vi "Process.vi"(8 "error in":errorcluster, 11 "Setting Database":refnum<class "Setting Database.lvclass">) -> (0 "error out":errorcluster, 3 "Setting Database out":refnum<class "Setting Database.lvclass">)   [LabVIEW 2019, in "Setting Database.lvclass"]
doc: "---------------------------------------------------------------\nJKI State Machine Objects™\nhttp://jki.net/state-machine-objects/\nCopyright (C) 2005-2015, JKI <info@jki.net>\nALL RIGHTS RESERVED"
uses:
  Setting Database.lvclass
  C:/Program Files (x86)/National Instruments/LabVIEW 2019/vi.lib/JKI/JKI SMO/SMO/SMO.lvclass
  <vilib>/JKI/JKI SMO/SMO/Typedefs/Parent Call--Enum.ctl
  Setting Database.lvclass/Setting Database.ctl
  ObjectSettings/ObjectSettings.lvclass/ObjectSettings.ctl
  Typedefs/PrivateEvents--Setting Database.Refresh.ctl
  <vilib>/JKI/JKI SMO/SMO/SMO.lvclass/SMO.ctl
  <vilib>/JKI/JKI SMO/SMO/Private/ReftoDVR--SMO.vi
  Dot Settings/Dot Settings.lvclass
  C:/Users/Albro/Documents/GitHub/AFM-Lithography/lvsrc/Classes/Settings/ObjectSettings/ObjectSettings.lvclass
  Funnel Settings/Funnel Settings.lvclass
  Rectangle Settings/Rectangle Settings.lvclass
  Path Settings/Path Settings.lvclass
  <vilib>/Utility/sysdir.llb/Get System Directory.vi
  Objects to GUIDs.vi
  <vilib>/JKI/JKI SMO/SMO/SMO.lvclass
  ObjectSettings/ObjectSettings.lvclass
  Identity/Identifier.lvclass
panel:
  # "For instructions on how to use the JKI State Machine Objects, examples and video tutorials, visit:\nhttp://jki.net/state-machine-objects/\n\nJKI State Machine Objects™\nhttp://jki.net/state-machine-objects/\nCopyright (C) 2005-2015, JKI <info@jki.net>\nALL RIGHTS RESERVED"
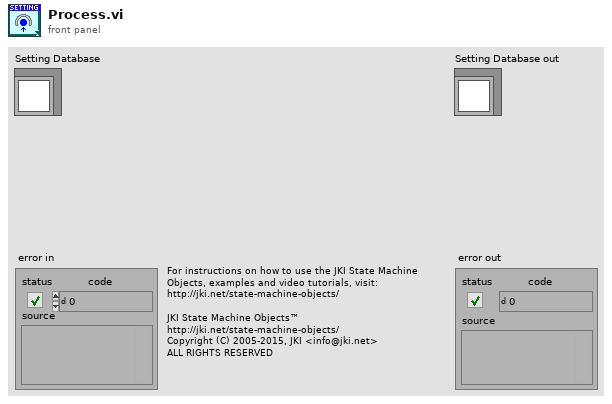
[diagram p1: front panel]
types:
  T1 = typedef "SMO.lvclass/Parent Call--Enum.ctl" = enum16{"Allows parent to run", "Does not request parent to run"}
  T2 = typedef "Setting Database.lvclass/PrivateEvents--Setting Database.Refresh.ctl" = cluster{"Paths":string[], "Rectangles":string[], "Funnels":string[], "Dots":string[]}
  T3 = enum32{"invalid app kind", "Development System", "Run Time System", "Student Edition", "Embedded LabVIEW", "Evaluation", "Custom"}
  T4 = enum32{"Invalid", "Standard", "Closed", "Hidden", "Minimized", "Maximized"}
  T5 = enum32{"Bad", "Idle", "Run top level", "Running"}
  T6 = cluster{"Core":cluster{"Current VI Reference":refnum<vi>, "Close Panel on Exit?":bool, "error":errorcluster}, "Self":refnum<class "Setting Database.lvclass">}
  T7 = typedef "Setting Database.lvclass/PrivateEvents--Setting Database.Remove From Group.ctl" = string
  T8 = typedef "Setting Database.lvclass/PrivateEvents--Setting Database.ChangeObjectEnable.ctl" = string
  T9 = typedef "Setting Database.lvclass/PrivateEvents--Setting Database.SetActivePath.ctl" = string
  T10 = cluster{"Path":string, "Funnel":string, "Rectangle":string, "Dot":string}
  T11 = typedef "Setting Database.lvclass/PrivateEvents--Setting Database.SetActiveDot.ctl" = string
  T12 = typedef "Setting Database.lvclass/PrivateEvents--Setting Database.SetActiveRectangle.ctl" = string
  T13 = typedef "Setting Database.lvclass/PrivateEvents--Setting Database.SetActiveFunnel.ctl" = string
  T14 = typedef "Setting Database.lvclass/PrivateEvents--Setting Database.UpdateActivePath.ctl" = refnum<class "Path Settings.lvclass">
  T15 = typedef "Setting Database.lvclass/PrivateEvents--Setting Database.UpdateActiveDot.ctl" = refnum<class "Dot Settings.lvclass">
  T16 = typedef "Setting Database.lvclass/PrivateEvents--Setting Database.UpdateActiveRectangle.ctl" = refnum<class "Rectangle Settings.lvclass">
  T17 = typedef "Setting Database.lvclass/PrivateEvents--Setting Database.UpdateActiveFunnel.ctl" = refnum<class "Funnel Settings.lvclass">
  T18 = cluster{"Current VI Reference":refnum<vi>, "Close Panel on Exit?":bool, "error":errorcluster}
  T19 = typedef "SMO.lvclass/Protected Events.ctl" = cluster{"StopProcesses":refnum<user-event>, "AbortProcesses":refnum<user-event>, "Config Changed":refnum<user-event>, "Dependency":refnum<user-event>}
  T20 = typedef "Setting Database.lvclass/PrivateEvents--Cluster.ctl" = cluster{"SetActivePath":refnum<user-event>, "UpdateActivePath":refnum<user-event>, "RefreshPaths":refnum<user-event>, "CopyActivePathToAll":refnum<user-event>, "SetActiveRectangle":refnum<user-event>, "UpdateActiveRectangle":refnum<user-event>, "CopyActiveRectangleToAll":refnum<user-event>, "SetActiveFunnel":refnum<user-event>, "UpdateActiveFunnel":refnum<user-event>, "CopyActiveFunnelToAll":refnum<user-event>, "SetDefaultPath":refnum<user-event>, "SetDefaultRectangle":refnum<user-event>, "SetDefaultFunnel":refnum<user-event>, "SetDefaultDot":refnum<user-event>, "SetActiveDot":refnum<user-event>, "UpdateActiveDot":refnum<user-event>, "CopyActiveDotToAll":refnum<user-event>, "ChangeObjectEnable":refnum<user-event>, "Create New Group":refnum<user-event>, "Add To Group":refnum<user-event>, "Remove From Group":refnum<user-event>, "Copy Settings To Group":refnum<user-event>}
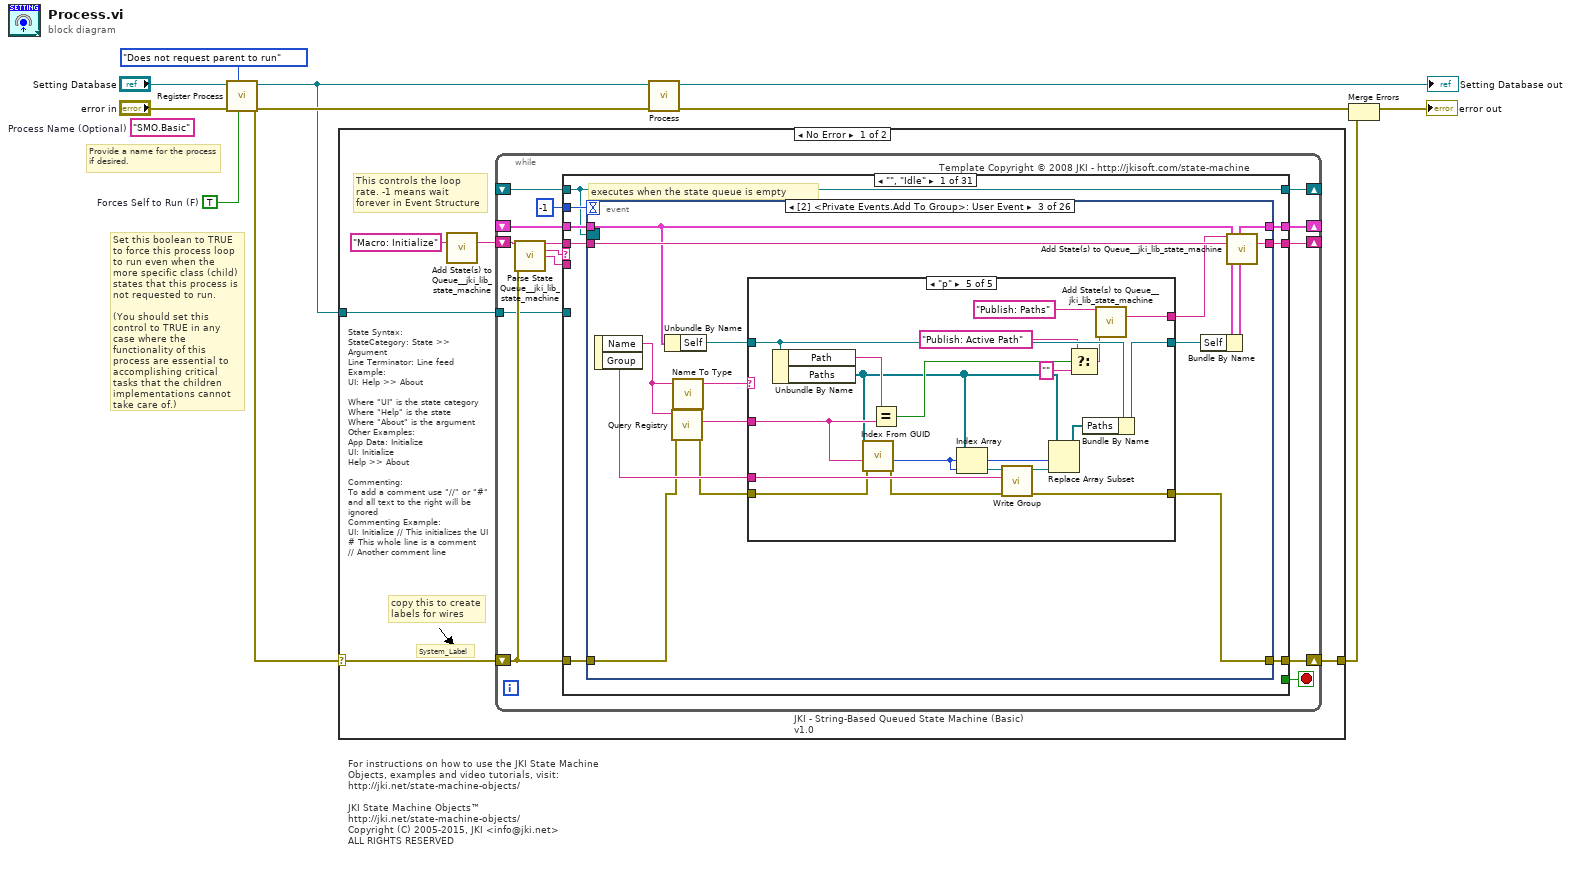
[diagram p0: block diagram]
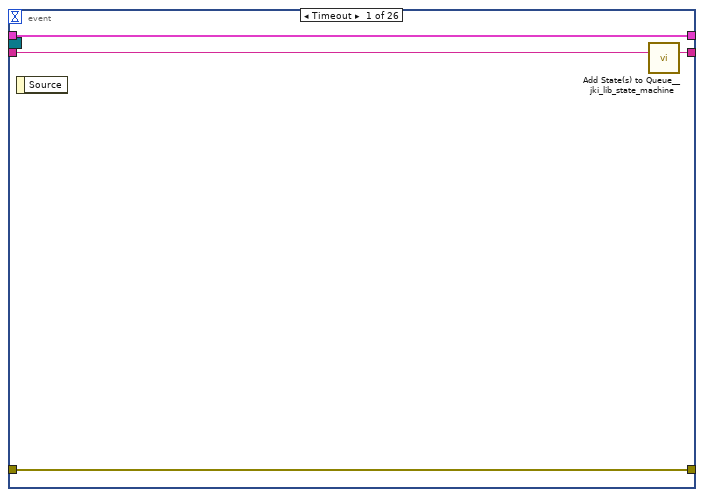
[diagram p2: hidden frame]
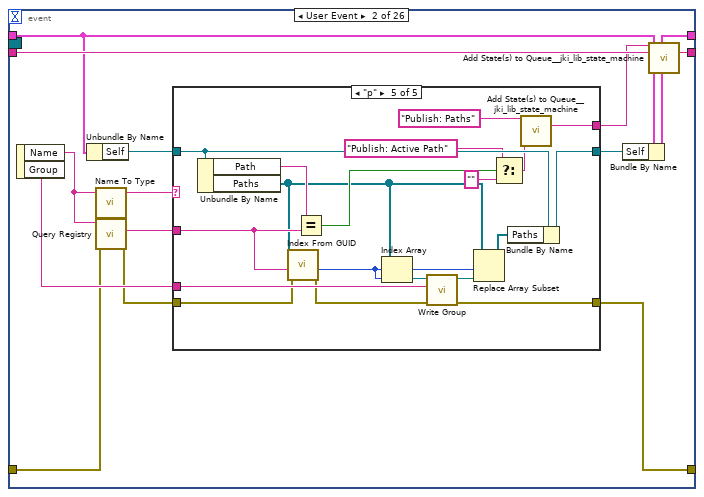
[diagram p3: hidden frame]
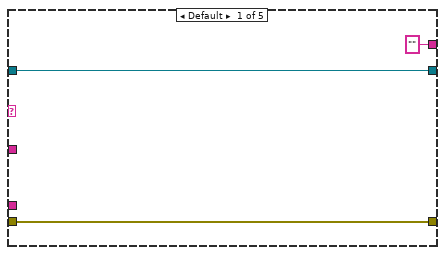
[diagram p4: hidden frame]
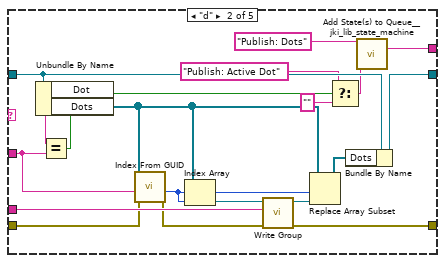
[diagram p5: hidden frame]
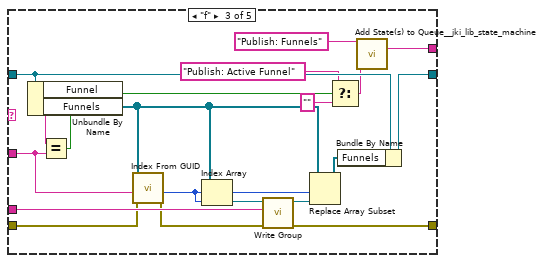
[diagram p6: hidden frame]
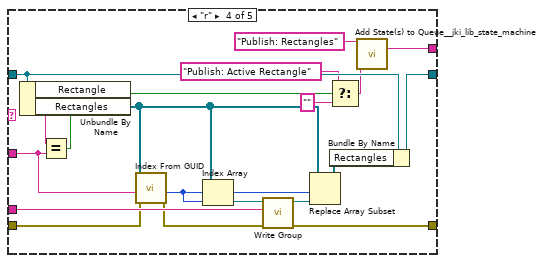
[diagram p7: hidden frame]
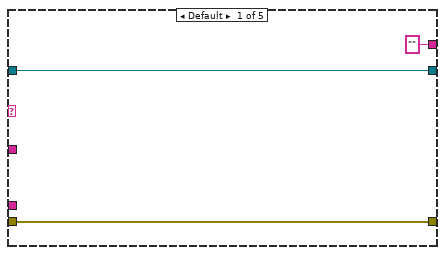
[diagram p8: hidden frame]
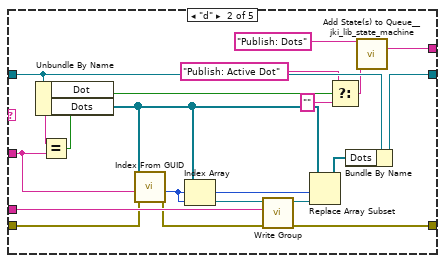
[diagram p9: hidden frame]
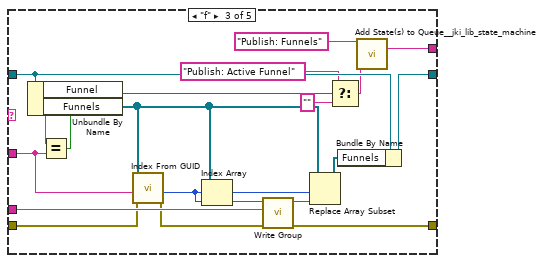
[diagram p10: hidden frame]
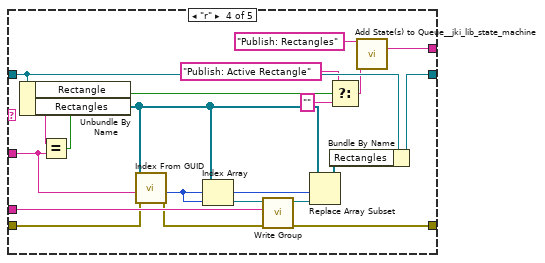
[diagram p11: hidden frame]
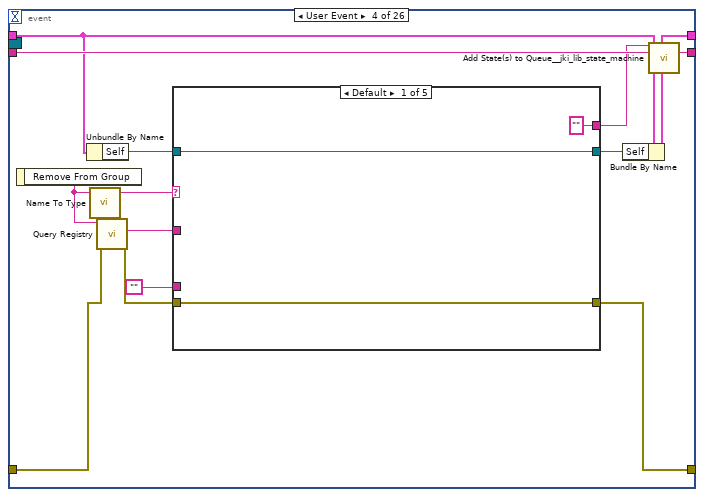
[diagram p12: hidden frame]
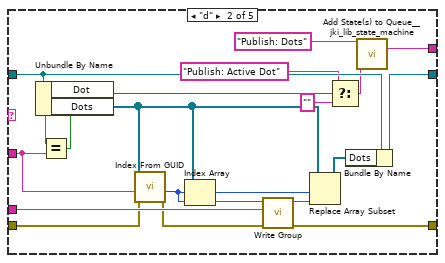
[diagram p13: hidden frame]
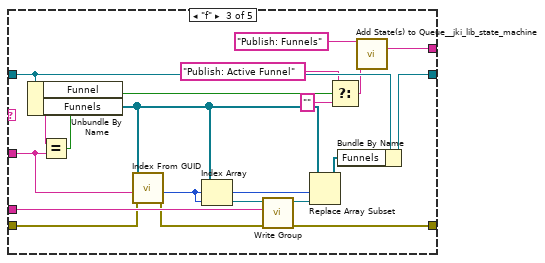
[diagram p14: hidden frame]
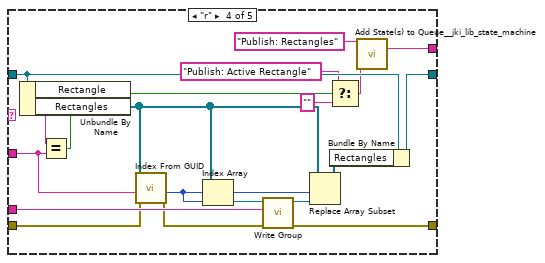
[diagram p15: hidden frame]
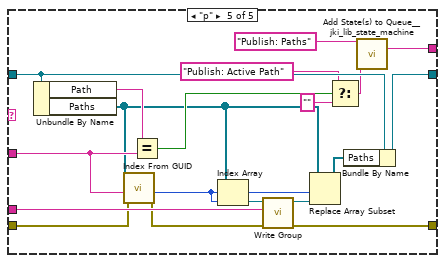
[diagram p16: hidden frame]
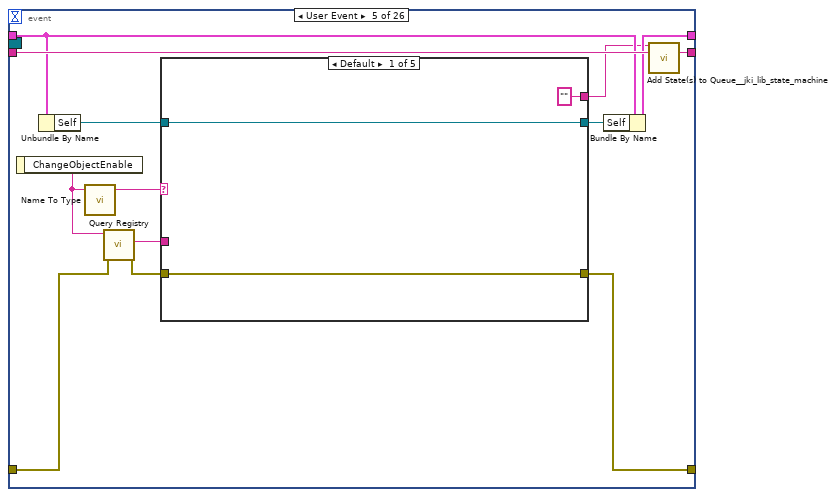
[diagram p17: hidden frame]
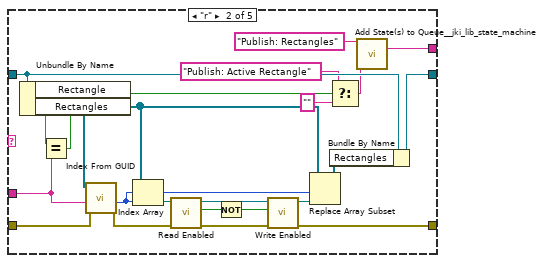
[diagram p18: hidden frame]
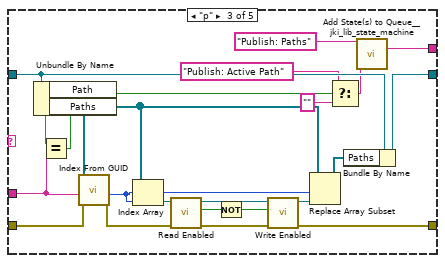
[diagram p19: hidden frame]
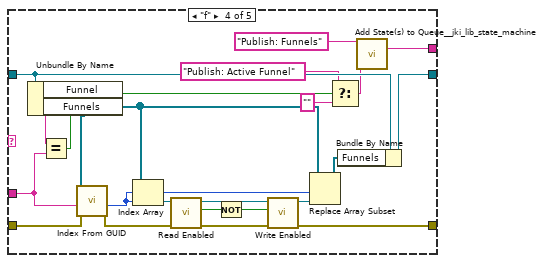
[diagram p20: hidden frame]
diagram:
  w1 = TRUE  # Forces Self to Run (F)
  (unwired) "SMO.Basic"  # Process Name (Optional)
  # "Provide a name for the process\nif desired."
  # "Set this boolean to TRUE to force this process loop to run even when the more specific class (child) states that this process is not requested to run.\n\n(You should set this control to TRUE in any case where the functionality of this process are essential to accomplishing critical tasks that the children implementations cannot take care of.)"
  # "For instructions on how to use the JKI State Machine Objects, examples and video tutorials, visit:\nhttp://jki.net/state-machine-objects/\n\nJKI State Machine Objects™\nhttp://jki.net/state-machine-objects/\nCopyright (C) 2005-2015, JKI <info@jki.net>\nALL RIGHTS RESERVED"
  n1 = call <vilib>:"Register Process.vi"("Forces Self to Run (F)"=w1, "Parent Call"=Parent_Call--Enum."Does not request parent to run", "error in (no error)"="error in", "SMO"="Setting Database") -> ("error out"=w8:errorcluster, "SMO out"=w4:refnum<class "Setting Database.lvclass">)  [unwired: 6 in]
  n2 = case shown="No Error" w8 {
    selector: w8 -> [w15 w1134]
    tunnel: w4 -> [w11 _]
    tunnel: [w14 w1134] -> w6
    frame No Error {
      # "State Syntax:\nStateCategory: State >> Argument\nLine Terminator: Line feed\nExample:\nUI: Help >> About\n\nWhere \"UI\" is the state category\nWhere \"Help\" is the state\nWhere \"About\" is the argument\nOther Examples:\nApp Data: Initialize\nUI: Initialize\nHelp >> About\n\nCommenting:\nTo add a comment use \"//\" or \"#\" and all text to the right will be ignored\nCommenting Example:\nUI: Initialize // This initializes the UI\n# This whole line is a comment\n// Another comment line"
      # "copy this to create labels for wires"
      # "This controls the loop rate. -1 means wait forever in Event Structure"
      # "System_Label"
      n3 = call <vilib>:"Add State(s) to Queue__jki_lib_state_machine.vi"("State(s) in (\"\")"="Macro: Initialize") -> ("States Out"=w13:string)  [unwired: 14 in]
      n4 = while "JKI - String-Based Queued State Machine (Basic) v1.0" {
        shift-right: [w21] -> _
        shift-left: _ -> [w20]
        shift-right: [w29] -> w14
        shift-left: w15 -> [w28]
        shift-right: [w23] -> _
        shift-left: w13 -> [w24]
        tunnel: w11 -> [w18]
        shift-right: [w17] -> _
        shift-left: _ -> [w16]
        stop <- w22 stop-if-true
        # "Template Copyright © 2008 JKI - http://jkisoft.com/state-machine"
        n5 = call <vilib>:"Parse State Queue__jki_lib_state_machine.vi"("State Queue"=w24, "Error In (no error)"=w28) -> ("Remaining States"=w26:string, "Current State"=w27:string, "Arguments"=w25:string)  [unwired: 11 in]
        n6 = case shown="\"\", \"Idle\"" w27 {
          selector: w27 -> [_ _ w817 _ _ _ _ _ _ _ _ _ _ _ _ _ _ _ _ _ _ _ _ _ _ _ _ _ _ _ _]
          tunnel: w26 -> [w35 w814 w821 w839 w850 w859 w864 w881 w889 w896 w902 w907 w913 w929 w962 w976 w990 w995 w1005 w1011 w1019 w1028 w1036 w1049 w1061 w1073 w1085 w1097 w1109 w1118 w1130]
          tunnel: w25 -> [_ _ _ _ _ _ _ _ _ _ _ _ w909 w925 _ _ _ _ _ _ _ _ _ _ _ _ _ _ _ _ _]
          tunnel: w20 -> [w33 w812 w819 w831 w846 w855 w862 w871 _ w893 w900 w905 w911 w927 w960 w973 w982 w993 w1002 w1009 w1017 w1026 w1032 w1045 w1057 w1069 w1081 w1093 w1105 w1111 w1127]
          tunnel: [w37 w815 w826 w840 w853 w860 w865 w870 w890 w897 w903 w908 w914 w930 w963 w977 w991 w996 w1006 w1012 w1023 w1030 w1037 w1039 w1051 w1063 w1076 w1087 w1099 w1120 w1132] -> w29
          tunnel: w28 -> [w36 w815 w825 w840 w854 _ w865 w868 w891 w898 w903 w908 w915 w931 w963 w977 w991 w996 w1007 w1012 w1024 w1030 w1037 w1038 w1050 w1067 w1080 w1086 w1098 w1119 w1131]
          tunnel: [w34 w813 w820 w838 w849 w858 w863 w880 w888 w895 w901 w906 w912 w928 w961 w975 w989 w994 w1004 w1010 w1018 w1027 w1035 w1048 w1060 w1072 w1084 w1096 w1108 w1117 w1129] -> w23
          tunnel: [_ _ _ _ _ TRUE _ _ _ _ _ _ _ _ _ _ _ _ _ _ _ _ _ _ _ _ _ _ _ _ _] -> w22
          tunnel: [w32 w812 w819 w837 w845 w855 w862 w872 w883 w893 w900 w905 w911 w927 w960 w973 w982 w993 w1002 w1009 w1017 w1026 w1033 w1046 w1058 w1070 w1082 w1094 w1106 w1112 w1126] -> w21
          tunnel: -1 ("Timeout") -> [w31 _ _ _ _ _ _ _ _ _ _ _ _ _ _ _ _ _ _ _ _ _ _ _ _ _ _ _ _ _ _]
          tunnel: w18 -> [_ _ _ _ _ _ _ _ w887 _ _ _ _ _ _ _ _ _ _ _ _ _ _ _ _ _ _ _ _ _ _]
          tunnel: [w30 w811 w816 w828 w848 w856 w861 w879 w886 w892 w899 w904 w910 w924 w959 w974 w983 w992 w1003 w1008 w1016 w1025 w1034 w1047 w1059 w1071 w1083 w1095 w1107 w1116 w1128] -> w17
          tunnel: w16 -> [w30 w811 w816 w828 w848 w856 w861 w879 w886 w892 w899 w904 w910 w924 w959 w974 w983 w992 w1003 w1008 _ w1025 w1034 w1047 w1059 w1071 w1083 w1095 w1107 w1116 w1128]
          frame "", "Idle" {
            # "executes when the state queue is empty"
            n7 = event shown="[2] <Private Events.Add To Group>: User Event" {
              selector: w30 -> [_ _ _ _ _ _ _ _ _ _ _ _ _ _ _ _ _ _ _ _ _ _ _ _ _ _]
              dyn-events: _ -> [_ _ _ _ _ _ _ _ _ _ _ _ _ _ _ _ _ _ _ _ _ _ _ _ _ _]
              timeout: w31 -> [_ _ _ _ _ _ _ _ _ _ _ _ _ _ _ _ _ _ _ _ _ _ _ _ _ _]
              tunnel: w35 -> [w40 w55 w148 w241 w333 w439 w448 w457 w466 w475 w489 w509 w643 w667 w691 w711 w723 w737 w751 w764 w774 w784 w794 w799 w804 w809]
              tunnel: [w39 w54 w147 w240 w332 w438 w447 w456 w465 w474 w488 w508 w642 w666 w690 w710 w722 w736 w750 w763 w773 w783 w793 w798 w803 w808] -> w34
              tunnel: w33 -> [w38 w51 w145 w238 w329 w436 w446 w455 w464 w473 w483 w505 w640 w664 w688 w708 w720 w734 w748 w761 w771 w781 w791 w797 w802 w807]
              tunnel: [w41 w49 w139 w228 w327 w431 w441 w453 w459 w468 w491 w511 w632 w657 w681 w701 w725 w739 w753 w756 w766 w776 w786 w800 w805 w810] -> w37
              tunnel: w36 -> [w41 w43 w135 w232 w321 w432 w440 w451 w458 w467 w490 w510 w633 w662 w675 w712 w724 w738 w752 w755 w767 w777 w787 w800 w805 w810]
              tunnel: [w38 w52 w146 w239 w330 w437 w446 w455 w464 w473 w484 w506 w641 w665 w689 w709 w721 w735 w749 w762 w772 w782 w792 w797 w802 w807] -> w32
              event Timeout {
                n8 = event-data() -> ()  [unwired: 1 in, 1 out]
                n9 = call <vilib>:"Add State(s) to Queue__jki_lib_state_machine.vi"("State(s) in (\"\")"=w40) -> ("States Out"=w39:string)  [unwired: 14 in]
              }
              event User Event {
                n10 = event-data() -> ("Name"=w45:string, "Group"=w47:string)  [unwired: 1 in]
                n11 = Unbundle By Name(w51) -> ("Self"=w53:refnum<class "Setting Database.lvclass">)
                n12 = call "Name To Type.vi"("Name"=w45) -> ("Type"=w46:string)  [unwired: 4 in]
                n13 = call "Query Registry.vi"("error in"=w43, "Name In"=w45) -> ("error out"=w42:errorcluster, "Alias"=w44:string)  [unwired: 6 in, 2 out]
                n14 = case shown="\"p\"" w46 {
                  tunnel: w53 -> [w58 w76 w95 w114 w133]
                  tunnel: [w58 w77 w96 w115 w134] -> w50
                  tunnel: [w57 w64 w83 w102 w123] -> w49
                  tunnel: w42 -> [w57 w59 w78 w97 w116]
                  tunnel: ["" ("States Out") w68 w87 w106 w127] -> w48
                  tunnel: w47 -> [_ w65 w84 w103 w124]
                  tunnel: w44 -> [_ w63 w81 w101 w120]
                  frame Default {
                  }
                  frame "d" {
                    n15 = Unbundle By Name(w76) -> ("Dot"=w74:string, "Dots"=w61:refnum<class "Dot Settings.lvclass">[])
                    n16 = Equal?(x=w74, y=w63) -> (x = y?=w70:bool)
                    n17 = call "Index From GUID.vi"("error in"=w59, "GUID"=w63, "Objects In"=w61) -> ("error out"=w60:errorcluster, "Index"=w62:i32)  [unwired: 5 in, 2 out]
                    n18 = Index Array(array=w61, index=w62) -> (element=w67:refnum<class "Dot Settings.lvclass">)
                    n19 = call-dynamic "Write Group.vi"("error in (no error)"=w60, "Group"=w65, "ObjectSettings in"=w67) -> ("error out"=w64:errorcluster, "ObjectSettings out"=w66:refnum<class "Dot Settings.lvclass">)  [unwired: 7 in]
                    n20 = Replace Array Subset(array=w61, new element=w66, index=w62) -> (w75:refnum<class "Dot Settings.lvclass">[])
                    n21 = Select(t="Publish: Active Dot", s=w70, f="") -> (s? t:f=w69:string)
                    n22 = Bundle By Name(cluster=w76, "Dots"=w75) -> (w77:refnum<class "Setting Database.lvclass">)
                    n23 = call <vilib>:"Add State(s) to Queue__jki_lib_state_machine.vi"("State(s) in Front (\"\")"="Publish: Dots", "State(s) in (\"\")"=w69) -> ("States Out"=w68:string)  [unwired: 13 in]
                  }
                  frame "f" {
                    n24 = Unbundle By Name(w95) -> ("Funnel"=w93:string, "Funnels"=w82:refnum<class "Funnel Settings.lvclass">[])
                    n25 = Equal?(x=w93, y=w81) -> (x = y?=w89:bool)
                    n26 = call "Index From GUID.vi"("error in"=w78, "GUID"=w81, "Objects In"=w82) -> ("error out"=w79:errorcluster, "Index"=w80:i32)  [unwired: 5 in, 2 out]
                    n27 = Index Array(array=w82, index=w80) -> (element=w86:refnum<class "Funnel Settings.lvclass">)
                    n28 = call-dynamic "Write Group.vi"("error in (no error)"=w79, "Group"=w84, "ObjectSettings in"=w86) -> ("error out"=w83:errorcluster, "ObjectSettings out"=w85:refnum<class "Funnel Settings.lvclass">)  [unwired: 7 in]
                    n29 = Replace Array Subset(array=w82, new element=w85, index=w80) -> (w94:refnum<class "Funnel Settings.lvclass">[])
                    n30 = Select(t="Publish: Active Funnel", s=w89, f="") -> (s? t:f=w88:string)
                    n31 = Bundle By Name(cluster=w95, "Funnels"=w94) -> (w96:refnum<class "Setting Database.lvclass">)
                    n32 = call <vilib>:"Add State(s) to Queue__jki_lib_state_machine.vi"("State(s) in Front (\"\")"="Publish: Funnels", "State(s) in (\"\")"=w88) -> ("States Out"=w87:string)  [unwired: 13 in]
                  }
                  frame "r" {
                    n33 = Unbundle By Name(w114) -> ("Rectangle"=w112:string, "Rectangles"=w99:refnum<class "Rectangle Settings.lvclass">[])
                    n34 = Equal?(x=w112, y=w101) -> (x = y?=w108:bool)
                    n35 = call "Index From GUID.vi"("error in"=w97, "GUID"=w101, "Objects In"=w99) -> ("error out"=w98:errorcluster, "Index"=w100:i32)  [unwired: 5 in, 2 out]
                    n36 = Index Array(array=w99, index=w100) -> (element=w105:refnum<class "Rectangle Settings.lvclass">)
                    n37 = call-dynamic "Write Group.vi"("error in (no error)"=w98, "Group"=w103, "ObjectSettings in"=w105) -> ("error out"=w102:errorcluster, "ObjectSettings out"=w104:refnum<class "Rectangle Settings.lvclass">)  [unwired: 7 in]
                    n38 = Replace Array Subset(array=w99, new element=w104, index=w100) -> (w113:refnum<class "Rectangle Settings.lvclass">[])
                    n39 = Select(t="Publish: Active Rectangle", s=w108, f="") -> (s? t:f=w107:string)
                    n40 = Bundle By Name(cluster=w114, "Rectangles"=w113) -> (w115:refnum<class "Setting Database.lvclass">)
                    n41 = call <vilib>:"Add State(s) to Queue__jki_lib_state_machine.vi"("State(s) in Front (\"\")"="Publish: Rectangles", "State(s) in (\"\")"=w107) -> ("States Out"=w106:string)  [unwired: 13 in]
                  }
                  frame "p" {
                    n42 = Unbundle By Name(w133) -> ("Path"=w122:string, "Paths"=w119:refnum<class "Path Settings.lvclass">[])
                    n43 = call "Index From GUID.vi"("error in"=w116, "GUID"=w120, "Objects In"=w119) -> ("error out"=w117:errorcluster, "Index"=w118:i32)  [unwired: 5 in, 2 out]
                    n44 = Equal?(x=w122, y=w120) -> (x = y?=w121:bool)
                    n45 = Index Array(array=w119, index=w118) -> (element=w126:refnum<class "Path Settings.lvclass">)
                    n46 = call-dynamic "Write Group.vi"("error in (no error)"=w117, "Group"=w124, "ObjectSettings in"=w126) -> ("error out"=w123:errorcluster, "ObjectSettings out"=w125:refnum<class "Path Settings.lvclass">)  [unwired: 7 in]
                    n47 = Replace Array Subset(array=w119, new element=w125, index=w118) -> (w132:refnum<class "Path Settings.lvclass">[])
                    n48 = Select(t="Publish: Active Path", s=w121, f="") -> (s? t:f=w128:string)
                    n49 = Bundle By Name(cluster=w133, "Paths"=w132) -> (w134:refnum<class "Setting Database.lvclass">)
                    n50 = call <vilib>:"Add State(s) to Queue__jki_lib_state_machine.vi"("State(s) in Front (\"\")"="Publish: Paths", "State(s) in (\"\")"=w128) -> ("States Out"=w127:string)  [unwired: 13 in]
                  }
                }
                n51 = Bundle By Name(cluster=w51, "Self"=w50) -> (w52:T6)
                n52 = call <vilib>:"Add State(s) to Queue__jki_lib_state_machine.vi"("State(s) in Front (\"\")"=w48, "State(s) in (\"\")"=w55) -> ("States Out"=w54:string)  [unwired: 13 in]
              }
              event User Event {
                n53 = event-data() -> ("Name"=w137:string, "Group"=w142:string)  [unwired: 1 in]
                n54 = Unbundle By Name(w145) -> ("Self"=w144:refnum<class "Setting Database.lvclass">)
                n55 = call "Query Registry.vi"("error in"=w135, "Name In"=w137) -> ("error out"=w136:errorcluster, "Alias"=w138:string)  [unwired: 6 in, 2 out]
                n56 = call "Name To Type.vi"("Name"=w137) -> ("Type"=w143:string)  [unwired: 4 in]
                n57 = case shown="\"p\"" w143 {
                  tunnel: w144 -> [w151 w169 w188 w207 w226]
                  tunnel: [w151 w170 w189 w208 w227] -> w140
                  tunnel: [w150 w157 w176 w195 w216] -> w139
                  tunnel: w136 -> [w150 w152 w171 w190 w209]
                  tunnel: ["" ("States Out") w161 w180 w199 w220] -> w141
                  tunnel: w142 -> [_ w158 w177 w196 w217]
                  tunnel: w138 -> [_ w156 w174 w194 w213]
                  frame Default {
                  }
                  frame "d" {
                    n58 = Unbundle By Name(w169) -> ("Dot"=w167:string, "Dots"=w154:refnum<class "Dot Settings.lvclass">[])
                    n59 = Equal?(x=w167, y=w156) -> (x = y?=w163:bool)
                    n60 = call "Index From GUID.vi"("error in"=w152, "GUID"=w156, "Objects In"=w154) -> ("error out"=w153:errorcluster, "Index"=w155:i32)  [unwired: 5 in, 2 out]
                    n61 = Index Array(array=w154, index=w155) -> (element=w160:refnum<class "Dot Settings.lvclass">)
                    n62 = call-dynamic "Write Group.vi"("error in (no error)"=w153, "Group"=w158, "ObjectSettings in"=w160) -> ("error out"=w157:errorcluster, "ObjectSettings out"=w159:refnum<class "Dot Settings.lvclass">)  [unwired: 7 in]
                    n63 = Replace Array Subset(array=w154, new element=w159, index=w155) -> (w168:refnum<class "Dot Settings.lvclass">[])
                    n64 = Select(t="Publish: Active Dot", s=w163, f="") -> (s? t:f=w162:string)
                    n65 = Bundle By Name(cluster=w169, "Dots"=w168) -> (w170:refnum<class "Setting Database.lvclass">)
                    n66 = call <vilib>:"Add State(s) to Queue__jki_lib_state_machine.vi"("State(s) in Front (\"\")"="Publish: Dots", "State(s) in (\"\")"=w162) -> ("States Out"=w161:string)  [unwired: 13 in]
                  }
                  frame "f" {
                    n67 = Unbundle By Name(w188) -> ("Funnel"=w186:string, "Funnels"=w175:refnum<class "Funnel Settings.lvclass">[])
                    n68 = Equal?(x=w186, y=w174) -> (x = y?=w182:bool)
                    n69 = call "Index From GUID.vi"("error in"=w171, "GUID"=w174, "Objects In"=w175) -> ("error out"=w172:errorcluster, "Index"=w173:i32)  [unwired: 5 in, 2 out]
                    n70 = Index Array(array=w175, index=w173) -> (element=w179:refnum<class "Funnel Settings.lvclass">)
                    n71 = call-dynamic "Write Group.vi"("error in (no error)"=w172, "Group"=w177, "ObjectSettings in"=w179) -> ("error out"=w176:errorcluster, "ObjectSettings out"=w178:refnum<class "Funnel Settings.lvclass">)  [unwired: 7 in]
                    n72 = Replace Array Subset(array=w175, new element=w178, index=w173) -> (w187:refnum<class "Funnel Settings.lvclass">[])
                    n73 = Select(t="Publish: Active Funnel", s=w182, f="") -> (s? t:f=w181:string)
                    n74 = Bundle By Name(cluster=w188, "Funnels"=w187) -> (w189:refnum<class "Setting Database.lvclass">)
                    n75 = call <vilib>:"Add State(s) to Queue__jki_lib_state_machine.vi"("State(s) in Front (\"\")"="Publish: Funnels", "State(s) in (\"\")"=w181) -> ("States Out"=w180:string)  [unwired: 13 in]
                  }
                  frame "r" {
                    n76 = Unbundle By Name(w207) -> ("Rectangle"=w205:string, "Rectangles"=w192:refnum<class "Rectangle Settings.lvclass">[])
                    n77 = Equal?(x=w205, y=w194) -> (x = y?=w201:bool)
                    n78 = call "Index From GUID.vi"("error in"=w190, "GUID"=w194, "Objects In"=w192) -> ("error out"=w191:errorcluster, "Index"=w193:i32)  [unwired: 5 in, 2 out]
                    n79 = Index Array(array=w192, index=w193) -> (element=w198:refnum<class "Rectangle Settings.lvclass">)
                    n80 = call-dynamic "Write Group.vi"("error in (no error)"=w191, "Group"=w196, "ObjectSettings in"=w198) -> ("error out"=w195:errorcluster, "ObjectSettings out"=w197:refnum<class "Rectangle Settings.lvclass">)  [unwired: 7 in]
                    n81 = Replace Array Subset(array=w192, new element=w197, index=w193) -> (w206:refnum<class "Rectangle Settings.lvclass">[])
                    n82 = Select(t="Publish: Active Rectangle", s=w201, f="") -> (s? t:f=w200:string)
                    n83 = Bundle By Name(cluster=w207, "Rectangles"=w206) -> (w208:refnum<class "Setting Database.lvclass">)
                    n84 = call <vilib>:"Add State(s) to Queue__jki_lib_state_machine.vi"("State(s) in Front (\"\")"="Publish: Rectangles", "State(s) in (\"\")"=w200) -> ("States Out"=w199:string)  [unwired: 13 in]
                  }
                  frame "p" {
                    n85 = Unbundle By Name(w226) -> ("Path"=w215:string, "Paths"=w212:refnum<class "Path Settings.lvclass">[])
                    n86 = call "Index From GUID.vi"("error in"=w209, "GUID"=w213, "Objects In"=w212) -> ("error out"=w210:errorcluster, "Index"=w211:i32)  [unwired: 5 in, 2 out]
                    n87 = Equal?(x=w215, y=w213) -> (x = y?=w214:bool)
                    n88 = Index Array(array=w212, index=w211) -> (element=w219:refnum<class "Path Settings.lvclass">)
                    n89 = call-dynamic "Write Group.vi"("error in (no error)"=w210, "Group"=w217, "ObjectSettings in"=w219) -> ("error out"=w216:errorcluster, "ObjectSettings out"=w218:refnum<class "Path Settings.lvclass">)  [unwired: 7 in]
                    n90 = Replace Array Subset(array=w212, new element=w218, index=w211) -> (w225:refnum<class "Path Settings.lvclass">[])
                    n91 = Select(t="Publish: Active Path", s=w214, f="") -> (s? t:f=w221:string)
                    n92 = Bundle By Name(cluster=w226, "Paths"=w225) -> (w227:refnum<class "Setting Database.lvclass">)
                    n93 = call <vilib>:"Add State(s) to Queue__jki_lib_state_machine.vi"("State(s) in Front (\"\")"="Publish: Paths", "State(s) in (\"\")"=w221) -> ("States Out"=w220:string)  [unwired: 13 in]
                  }
                }
                n94 = Bundle By Name(cluster=w145, "Self"=w140) -> (w146:T6)
                n95 = call <vilib>:"Add State(s) to Queue__jki_lib_state_machine.vi"("State(s) in Front (\"\")"=w141, "State(s) in (\"\")"=w148) -> ("States Out"=w147:string)  [unwired: 13 in]
              }
              event User Event {
                n96 = event-data() -> ("Remove From Group"=w231:T7)  [unwired: 1 in]
                n97 = Unbundle By Name(w238) -> ("Self"=w234:refnum<class "Setting Database.lvclass">)
                n98 = call "Name To Type.vi"("Name"=w231) -> ("Type"=w233:string)  [unwired: 4 in]
                n99 = call "Query Registry.vi"("error in"=w232, "Name In"=w231) -> ("error out"=w229:errorcluster, "Alias"=w237:string)  [unwired: 6 in, 2 out]
                n100 = case shown="Default" w233 {
                  tunnel: w234 -> [w244 w262 w281 w300 w319]
                  tunnel: [w244 w263 w282 w301 w320] -> w235
                  tunnel: [w243 w250 w269 w288 w309] -> w228
                  tunnel: w229 -> [w243 w245 w264 w283 w302]
                  tunnel: ["" ("States Out") w254 w273 w292 w313] -> w236
                  tunnel: "" -> [_ w251 w270 w289 w310]
                  tunnel: w237 -> [_ w249 w267 w287 w306]
                  frame Default {
                  }
                  frame "d" {
                    n101 = Unbundle By Name(w262) -> ("Dot"=w260:string, "Dots"=w247:refnum<class "Dot Settings.lvclass">[])
                    n102 = Equal?(x=w260, y=w249) -> (x = y?=w256:bool)
                    n103 = call "Index From GUID.vi"("error in"=w245, "GUID"=w249, "Objects In"=w247) -> ("error out"=w246:errorcluster, "Index"=w248:i32)  [unwired: 5 in, 2 out]
                    n104 = Index Array(array=w247, index=w248) -> (element=w253:refnum<class "Dot Settings.lvclass">)
                    n105 = call-dynamic "Write Group.vi"("error in (no error)"=w246, "Group"=w251, "ObjectSettings in"=w253) -> ("error out"=w250:errorcluster, "ObjectSettings out"=w252:refnum<class "Dot Settings.lvclass">)  [unwired: 7 in]
                    n106 = Replace Array Subset(array=w247, new element=w252, index=w248) -> (w261:refnum<class "Dot Settings.lvclass">[])
                    n107 = Select(t="Publish: Active Dot", s=w256, f="") -> (s? t:f=w255:string)
                    n108 = Bundle By Name(cluster=w262, "Dots"=w261) -> (w263:refnum<class "Setting Database.lvclass">)
                    n109 = call <vilib>:"Add State(s) to Queue__jki_lib_state_machine.vi"("State(s) in Front (\"\")"="Publish: Dots", "State(s) in (\"\")"=w255) -> ("States Out"=w254:string)  [unwired: 13 in]
                  }
                  frame "f" {
                    n110 = Unbundle By Name(w281) -> ("Funnel"=w279:string, "Funnels"=w268:refnum<class "Funnel Settings.lvclass">[])
                    n111 = Equal?(x=w279, y=w267) -> (x = y?=w275:bool)
                    n112 = call "Index From GUID.vi"("error in"=w264, "GUID"=w267, "Objects In"=w268) -> ("error out"=w265:errorcluster, "Index"=w266:i32)  [unwired: 5 in, 2 out]
                    n113 = Index Array(array=w268, index=w266) -> (element=w272:refnum<class "Funnel Settings.lvclass">)
                    n114 = call-dynamic "Write Group.vi"("error in (no error)"=w265, "Group"=w270, "ObjectSettings in"=w272) -> ("error out"=w269:errorcluster, "ObjectSettings out"=w271:refnum<class "Funnel Settings.lvclass">)  [unwired: 7 in]
                    n115 = Replace Array Subset(array=w268, new element=w271, index=w266) -> (w280:refnum<class "Funnel Settings.lvclass">[])
                    n116 = Select(t="Publish: Active Funnel", s=w275, f="") -> (s? t:f=w274:string)
                    n117 = Bundle By Name(cluster=w281, "Funnels"=w280) -> (w282:refnum<class "Setting Database.lvclass">)
                    n118 = call <vilib>:"Add State(s) to Queue__jki_lib_state_machine.vi"("State(s) in Front (\"\")"="Publish: Funnels", "State(s) in (\"\")"=w274) -> ("States Out"=w273:string)  [unwired: 13 in]
                  }
                  frame "r" {
                    n119 = Unbundle By Name(w300) -> ("Rectangle"=w298:string, "Rectangles"=w285:refnum<class "Rectangle Settings.lvclass">[])
                    n120 = Equal?(x=w298, y=w287) -> (x = y?=w294:bool)
                    n121 = call "Index From GUID.vi"("error in"=w283, "GUID"=w287, "Objects In"=w285) -> ("error out"=w284:errorcluster, "Index"=w286:i32)  [unwired: 5 in, 2 out]
                    n122 = Index Array(array=w285, index=w286) -> (element=w291:refnum<class "Rectangle Settings.lvclass">)
                    n123 = call-dynamic "Write Group.vi"("error in (no error)"=w284, "Group"=w289, "ObjectSettings in"=w291) -> ("error out"=w288:errorcluster, "ObjectSettings out"=w290:refnum<class "Rectangle Settings.lvclass">)  [unwired: 7 in]
                    n124 = Replace Array Subset(array=w285, new element=w290, index=w286) -> (w299:refnum<class "Rectangle Settings.lvclass">[])
                    n125 = Select(t="Publish: Active Rectangle", s=w294, f="") -> (s? t:f=w293:string)
                    n126 = Bundle By Name(cluster=w300, "Rectangles"=w299) -> (w301:refnum<class "Setting Database.lvclass">)
                    n127 = call <vilib>:"Add State(s) to Queue__jki_lib_state_machine.vi"("State(s) in Front (\"\")"="Publish: Rectangles", "State(s) in (\"\")"=w293) -> ("States Out"=w292:string)  [unwired: 13 in]
                  }
                  frame "p" {
                    n128 = Unbundle By Name(w319) -> ("Path"=w308:string, "Paths"=w305:refnum<class "Path Settings.lvclass">[])
                    n129 = call "Index From GUID.vi"("error in"=w302, "GUID"=w306, "Objects In"=w305) -> ("error out"=w303:errorcluster, "Index"=w304:i32)  [unwired: 5 in, 2 out]
                    n130 = Equal?(x=w308, y=w306) -> (x = y?=w307:bool)
                    n131 = Index Array(array=w305, index=w304) -> (element=w312:refnum<class "Path Settings.lvclass">)
                    n132 = call-dynamic "Write Group.vi"("error in (no error)"=w303, "Group"=w310, "ObjectSettings in"=w312) -> ("error out"=w309:errorcluster, "ObjectSettings out"=w311:refnum<class "Path Settings.lvclass">)  [unwired: 7 in]
                    n133 = Replace Array Subset(array=w305, new element=w311, index=w304) -> (w318:refnum<class "Path Settings.lvclass">[])
                    n134 = Select(t="Publish: Active Path", s=w307, f="") -> (s? t:f=w314:string)
                    n135 = Bundle By Name(cluster=w319, "Paths"=w318) -> (w320:refnum<class "Setting Database.lvclass">)
                    n136 = call <vilib>:"Add State(s) to Queue__jki_lib_state_machine.vi"("State(s) in Front (\"\")"="Publish: Paths", "State(s) in (\"\")"=w314) -> ("States Out"=w313:string)  [unwired: 13 in]
                  }
                }
                n137 = Bundle By Name(cluster=w238, "Self"=w235) -> (w239:T6)
                n138 = call <vilib>:"Add State(s) to Queue__jki_lib_state_machine.vi"("State(s) in Front (\"\")"=w236, "State(s) in (\"\")"=w241) -> ("States Out"=w240:string)  [unwired: 13 in]
              }
              event User Event {
                n139 = event-data() -> ("ChangeObjectEnable"=w324:T8)  [unwired: 1 in]
                n140 = Unbundle By Name(w329) -> ("Self"=w331:refnum<class "Setting Database.lvclass">)
                n141 = call "Name To Type.vi"("Name"=w324) -> ("Type"=w325:string)  [unwired: 4 in]
                n142 = call "Query Registry.vi"("error in"=w321, "Name In"=w324) -> ("error out"=w322:errorcluster, "Alias"=w323:string)  [unwired: 6 in, 2 out]
                n143 = case shown="Default" w325 {
                  tunnel: w331 -> [w336 w354 w376 w398 w420]
                  tunnel: [w336 w355 w377 w399 w421] -> w328
                  tunnel: [w335 w349 w371 w393 w415] -> w327
                  tunnel: w322 -> [w335 w338 w360 w381 w403]
                  tunnel: ["" ("States Out") w342 w364 w386 w408] -> w326
                  tunnel: w323 -> [_ w337 w362 w384 w407]
                  frame Default {
                  }
                  frame "r" {
                    n144 = Unbundle By Name(w354) -> ("Rectangle"=w348:string, "Rectangles"=w341:refnum<class "Rectangle Settings.lvclass">[])
                    n145 = Equal?(x=w348, y=w337) -> (x = y?=w344:bool)
                    n146 = call "Index From GUID.vi"("error in"=w338, "GUID"=w337, "Objects In"=w341) -> ("error out"=w339:errorcluster, "Index"=w340:i32)  [unwired: 5 in, 2 out]
                    n147 = Index Array(array=w341, index=w340) -> (element=w358:refnum<class "Rectangle Settings.lvclass">)
                    n148 = call "Read Enabled.vi"("error in (no error)"=w339, "ObjectSettings in"=w358) -> ("error out"=w350:errorcluster, "Enabled"=w352:bool, "ObjectSettings out"=w357:refnum<class "Rectangle Settings.lvclass">)  [unwired: 7 in]
                    n149 = Not(x=w352) -> (.not. x?=w351:bool)
                    n150 = call "Write Enabled.vi"("error in (no error)"=w350, "Enabled"=w351, "ObjectSettings in"=w357) -> ("error out"=w349:errorcluster, "ObjectSettings out"=w356:refnum<class "Rectangle Settings.lvclass">)  [unwired: 7 in]
                    n151 = Replace Array Subset(array=w341, new element=w356, index=w340) -> (w353:refnum<class "Rectangle Settings.lvclass">[])
                    n152 = Select(t="Publish: Active Rectangle", s=w344, f="") -> (s? t:f=w343:string)
                    n153 = Bundle By Name(cluster=w354, "Rectangles"=w353) -> (w355:refnum<class "Setting Database.lvclass">)
                    n154 = call <vilib>:"Add State(s) to Queue__jki_lib_state_machine.vi"("State(s) in Front (\"\")"="Publish: Rectangles", "State(s) in (\"\")"=w343) -> ("States Out"=w342:string)  [unwired: 13 in]
                  }
                  frame "p" {
                    n155 = Unbundle By Name(w376) -> ("Path"=w370:string, "Paths"=w363:refnum<class "Path Settings.lvclass">[])
                    n156 = Equal?(x=w370, y=w362) -> (x = y?=w366:bool)
                    n157 = call "Index From GUID.vi"("error in"=w360, "GUID"=w362, "Objects In"=w363) -> ("error out"=w361:errorcluster, "Index"=w359:i32)  [unwired: 5 in, 2 out]
                    n158 = Index Array(array=w363, index=w359) -> (element=w380:refnum<class "Path Settings.lvclass">)
                    n159 = call "Read Enabled.vi"("error in (no error)"=w361, "ObjectSettings in"=w380) -> ("error out"=w372:errorcluster, "Enabled"=w374:bool, "ObjectSettings out"=w379:refnum<class "Path Settings.lvclass">)  [unwired: 7 in]
                    n160 = Not(x=w374) -> (.not. x?=w373:bool)
                    n161 = call "Write Enabled.vi"("error in (no error)"=w372, "Enabled"=w373, "ObjectSettings in"=w379) -> ("error out"=w371:errorcluster, "ObjectSettings out"=w378:refnum<class "Path Settings.lvclass">)  [unwired: 7 in]
                    n162 = Replace Array Subset(array=w363, new element=w378, index=w359) -> (w375:refnum<class "Path Settings.lvclass">[])
                    n163 = Select(t="Publish: Active Path", s=w366, f="") -> (s? t:f=w365:string)
                    n164 = Bundle By Name(cluster=w376, "Paths"=w375) -> (w377:refnum<class "Setting Database.lvclass">)
                    n165 = call <vilib>:"Add State(s) to Queue__jki_lib_state_machine.vi"("State(s) in Front (\"\")"="Publish: Paths", "State(s) in (\"\")"=w365) -> ("States Out"=w364:string)  [unwired: 13 in]
                  }
                  frame "f" {
                    n166 = Unbundle By Name(w398) -> ("Funnel"=w392:string, "Funnels"=w385:refnum<class "Funnel Settings.lvclass">[])
                    n167 = Equal?(x=w392, y=w384) -> (x = y?=w388:bool)
                    n168 = call "Index From GUID.vi"("error in"=w381, "GUID"=w384, "Objects In"=w385) -> ("error out"=w382:errorcluster, "Index"=w383:i32)  [unwired: 5 in, 2 out]
                    n169 = Index Array(array=w385, index=w383) -> (element=w402:refnum<class "Funnel Settings.lvclass">)
                    n170 = call "Read Enabled.vi"("error in (no error)"=w382, "ObjectSettings in"=w402) -> ("error out"=w394:errorcluster, "Enabled"=w396:bool, "ObjectSettings out"=w401:refnum<class "Funnel Settings.lvclass">)  [unwired: 7 in]
                    n171 = Not(x=w396) -> (.not. x?=w395:bool)
                    n172 = call "Write Enabled.vi"("error in (no error)"=w394, "Enabled"=w395, "ObjectSettings in"=w401) -> ("error out"=w393:errorcluster, "ObjectSettings out"=w400:refnum<class "Funnel Settings.lvclass">)  [unwired: 7 in]
                    n173 = Replace Array Subset(array=w385, new element=w400, index=w383) -> (w397:refnum<class "Funnel Settings.lvclass">[])
                    n174 = Select(t="Publish: Active Funnel", s=w388, f="") -> (s? t:f=w387:string)
                    n175 = Bundle By Name(cluster=w398, "Funnels"=w397) -> (w399:refnum<class "Setting Database.lvclass">)
                    n176 = call <vilib>:"Add State(s) to Queue__jki_lib_state_machine.vi"("State(s) in Front (\"\")"="Publish: Funnels", "State(s) in (\"\")"=w387) -> ("States Out"=w386:string)  [unwired: 13 in]
                  }
                  frame "d" {
                    n177 = Unbundle By Name(w420) -> ("Dot"=w414:string, "Dots"=w406:refnum<class "Dot Settings.lvclass">[])
                    n178 = Equal?(x=w414, y=w407) -> (x = y?=w410:bool)
                    n179 = call "Index From GUID.vi"("error in"=w403, "GUID"=w407, "Objects In"=w406) -> ("error out"=w404:errorcluster, "Index"=w405:i32)  [unwired: 5 in, 2 out]
                    n180 = Index Array(array=w406, index=w405) -> (element=w424:refnum<class "Dot Settings.lvclass">)
                    n181 = call "Read Enabled.vi"("error in (no error)"=w404, "ObjectSettings in"=w424) -> ("error out"=w416:errorcluster, "Enabled"=w418:bool, "ObjectSettings out"=w423:refnum<class "Dot Settings.lvclass">)  [unwired: 7 in]
                    n182 = Not(x=w418) -> (.not. x?=w417:bool)
                    n183 = call "Write Enabled.vi"("error in (no error)"=w416, "Enabled"=w417, "ObjectSettings in"=w423) -> ("error out"=w415:errorcluster, "ObjectSettings out"=w422:refnum<class "Dot Settings.lvclass">)  [unwired: 7 in]
                    n184 = Replace Array Subset(array=w406, new element=w422, index=w405) -> (w419:refnum<class "Dot Settings.lvclass">[])
                    n185 = Select(t="Publish: Active Dot", s=w410, f="") -> (s? t:f=w409:string)
                    n186 = Bundle By Name(cluster=w420, "Dots"=w419) -> (w421:refnum<class "Setting Database.lvclass">)
                    n187 = call <vilib>:"Add State(s) to Queue__jki_lib_state_machine.vi"("State(s) in Front (\"\")"="Publish: Dots", "State(s) in (\"\")"=w409) -> ("States Out"=w408:string)  [unwired: 13 in]
                  }
                }
                n188 = Bundle By Name(cluster=w329, "Self"=w328) -> (w330:T6)
                n189 = call <vilib>:"Add State(s) to Queue__jki_lib_state_machine.vi"("State(s) in Front (\"\")"=w326, "State(s) in (\"\")"=w333) -> ("States Out"=w332:string)  [unwired: 13 in]
              }
              event User Event {
                # "Basically a message broker that manages settings as well"
                # "#todo\nDocument this"
                n190 = event-data() -> ("Paths"=w430:string[], "Rectangles"=w428:string[], "Funnels"=w427:string[], "Dots"=w425:string[])  [unwired: 1 in]
                n191 = Bundle By Name(cluster=T2 {"Paths"=[], "Rectangles"=[], "Funnels"=[], "Dots"=[]} ("Refresh"), "Paths"=w430, "Rectangles"=w428, "Funnels"=w427, "Dots"=w425) -> (w426:T2)
                n192 = Unbundle By Name(w436) -> ("Self"=w434:refnum<class "Setting Database.lvclass">)
                n193 = call "RefreshAllObjects.vi"("error in (no error)"=w432, "Refresh"=w426, "Setting Database in"=w434) -> ("error out"=w431:errorcluster, "Setting Database out"=w433:refnum<class "Setting Database.lvclass">)  [unwired: 7 in]
                n194 = Bundle By Name(cluster=w436, "Self"=w433) -> (w437:T6)
                n195 = call <vilib>:"Add State(s) to Queue__jki_lib_state_machine.vi"("State(s) in Front (\"\")"="Publish: Paths\nPublish: Funnels\nPublish: Rectangles\nPublish: Dots\nPublish: Active Path\nPublish: Active Funnel\nPublish: Active Rectangle\nPublish: Active Dot", "State(s) in (\"\")"=w439) -> ("States Out"=w438:string)  [unwired: 13 in]
              }
              event User Event {
                # "Here we would write the current value to file as the default value"
                n196 = event-data() -> ()  [unwired: 1 in, 1 out]
                n197 = Unbundle By Name(w446) -> ("Self"=w445:refnum<class "Setting Database.lvclass">)
                n198 = call "Read Active Rectangle.vi"("error in (no error)"=w440, "Setting Database in"=w445) -> ("error out"=w442:errorcluster, "Active Rectangle"=w444:refnum<class "Rectangle Settings.lvclass">)  [unwired: 7 in, 1 out]
                n199 = call "Base INI Folder Path.vi"() -> ("Base Path"=w443:path)  [unwired: 11 in]
                n200 = call-dynamic "Write Default to File.vi"("error in (no error)"=w442, "Path"=w443, "Rectangle Settings in"=w444) -> ("error out"=w441:errorcluster)  [unwired: 7 in, 1 out]
                n201 = call <vilib>:"Add State(s) to Queue__jki_lib_state_machine.vi"("State(s) in (\"\")"=w448) -> ("States Out"=w447:string)  [unwired: 14 in]
              }
              event User Event {
                # "Here we would write the current value to file as the default value"
                n202 = event-data() -> ()  [unwired: 1 in, 5 out]
                n203 = Unbundle By Name(w455) -> ("Self"=w452:refnum<class "Setting Database.lvclass">)
                n204 = call "Read Active Dot.vi"("error in (no error)"=w451, "Setting Database in"=w452) -> ("error out"=w450:errorcluster, "Active Dot"=w449:refnum<class "Dot Settings.lvclass">)  [unwired: 7 in, 1 out]
                n205 = call "Base INI Folder Path.vi"() -> ("Base Path"=w454:path)  [unwired: 11 in]
                n206 = call-dynamic "Write Default to File.vi"("error in (no error)"=w450, "Path"=w454, "Dot Settings in"=w449) -> ("error out"=w453:errorcluster)  [unwired: 7 in, 1 out]
                n207 = call <vilib>:"Add State(s) to Queue__jki_lib_state_machine.vi"("State(s) in (\"\")"=w457) -> ("States Out"=w456:string)  [unwired: 14 in]
              }
              event User Event {
                # "Here we would write the current value to file as the default value"
                n208 = event-data() -> ()  [unwired: 1 in, 5 out]
                n209 = Unbundle By Name(w464) -> ("Self"=w463:refnum<class "Setting Database.lvclass">)
                n210 = call "Read Active Path.vi"("error in (no error)"=w458, "Setting Database in"=w463) -> ("error out"=w460:errorcluster, "Path Settings.lvclass"=w462:refnum<class "Path Settings.lvclass">)  [unwired: 7 in, 1 out]
                n211 = call "Base INI Folder Path.vi"() -> ("Base Path"=w461:path)  [unwired: 11 in]
                n212 = call-dynamic "Write Default to File.vi"("error in (no error)"=w460, "Path"=w461, "Path Settings in"=w462) -> ("error out"=w459:errorcluster)  [unwired: 7 in, 1 out]
                n213 = call <vilib>:"Add State(s) to Queue__jki_lib_state_machine.vi"("State(s) in (\"\")"=w466) -> ("States Out"=w465:string)  [unwired: 14 in]
              }
              event User Event {
                # "Here we would write the current value to file as the default value"
                n214 = event-data() -> ()  [unwired: 1 in, 5 out]
                n215 = Unbundle By Name(w473) -> ("Self"=w472:refnum<class "Setting Database.lvclass">)
                n216 = call "Read Active Funnel.vi"("error in (no error)"=w467, "Setting Database in"=w472) -> ("error out"=w469:errorcluster, "Active Funnel"=w471:refnum<class "Funnel Settings.lvclass">)  [unwired: 7 in, 1 out]
                n217 = call "Base INI Folder Path.vi"() -> ("Base Path"=w470:path)  [unwired: 11 in]
                n218 = call-dynamic "Write Default to File.vi"("error in (no error)"=w469, "Path"=w470, "Funnel Settings in"=w471) -> ("error out"=w468:errorcluster)  [unwired: 7 in, 1 out]
                n219 = call <vilib>:"Add State(s) to Queue__jki_lib_state_machine.vi"("State(s) in (\"\")"=w475) -> ("States Out"=w474:string)  [unwired: 14 in]
              }
              event User Event {
                n220 = event-data() -> ()  [unwired: 1 in, 1 out]
                n221 = Unbundle By Name(w483) -> ("Self"=w487:refnum<class "Setting Database.lvclass">)
                n222 = call "Read Paths.vi"("error in (no error)"=w490, "Setting Database in"=w487) -> ("error out"=w492:errorcluster, "Paths"=w476:refnum<class "Path Settings.lvclass">[], "Setting Database out"=w486:refnum<class "Setting Database.lvclass">)  [unwired: 7 in]
                n223 = call "Read Active Path.vi"("error in (no error)"=w492, "Setting Database in"=w486) -> ("error out"=w480:errorcluster, "Path Settings.lvclass"=w477:refnum<class "Path Settings.lvclass">, "Setting Database out"=w485:refnum<class "Setting Database.lvclass">)  [unwired: 7 in]
                n224 = for {
                  shift-right: [w495] -> w479
                  shift-left: w480 -> [w497]
                  tunnel: [w496] -> w478 mode=indexing
                  tunnel: w477 -> [w494]
                  tunnel: w476 -> [w493] mode=indexing
                  n225 = call-dynamic "Read GUID.vi"("error in (no error)"=w497, "ObjectSettings in"=w493) -> ("error out"=w498:errorcluster, "GUID"=w499:string)  [unwired: 7 in, 1 out]
                  n226 = call-dynamic "Write GUID.vi"("error in (no error)"=w498, "GUID"=w499, "ObjectSettings in"=w494) -> ("error out"=w495:errorcluster, "ObjectSettings out"=w496:refnum<class "Path Settings.lvclass">)  [unwired: 7 in]
                }
                n227 = call "Write Paths.vi"("error in (no error)"=w479, "Paths"=w478, "Setting Database in"=w485) -> ("error out"=w491:errorcluster, "Setting Database out"=w482:refnum<class "Setting Database.lvclass">)  [unwired: 7 in]
                n228 = Bundle By Name(cluster=w483, "Self"=w482) -> (w484:T6)
                n229 = call <vilib>:"Add State(s) to Queue__jki_lib_state_machine.vi"("State(s) in Front (\"\")"="Publish: Paths", "State(s) in (\"\")"=w489) -> ("States Out"=w488:string)  [unwired: 13 in]
              }
              event User Event {
                n230 = event-data() -> ("Group"=w501:string, "Name"=w503:string)  [unwired: 1 in]
                n231 = call "Name To Type.vi"("Name"=w503) -> ("Type"=w502:string)  [unwired: 4 in]
                n232 = Unbundle By Name(w505) -> ("Self"=w507:refnum<class "Setting Database.lvclass">)
                n233 = case shown="\"d\"" w502 {
                  tunnel: [w514 w517 w544 w573 w600] -> w511
                  tunnel: w510 -> [w514 w516 w547 w579 w608]
                  tunnel: w507 -> [w513 w527 w555 w580 w611]
                  tunnel: [w513 w524 w553 w572 w604] -> w504
                  tunnel: w501 -> [_ w520 w556 w584 w612]
                  tunnel: ["" "Publish: Paths" "Publish: Rectangles" "Publish: Funnels" "Publish: Dots"] -> w500
                  frame Default {
                  }
                  frame "p" {
                    n234 = call "Read Paths.vi"("error in (no error)"=w516, "Setting Database in"=w527) -> ("error out"=w528:errorcluster, "Paths"=w522:refnum<class "Path Settings.lvclass">[], "Setting Database out"=w526:refnum<class "Setting Database.lvclass">)  [unwired: 7 in]
                    n235 = call "Read Active Path.vi"("error in (no error)"=w528, "Setting Database in"=w526) -> ("error out"=w519:errorcluster, "Path Settings.lvclass"=w521:refnum<class "Path Settings.lvclass">, "Setting Database out"=w525:refnum<class "Setting Database.lvclass">)  [unwired: 7 in]
                    n236 = for {
                      shift-right: [w540] -> w518
                      shift-left: w519 -> [w536]
                      tunnel: [w529] -> w523 mode=indexing
                      tunnel: w521 -> [w539]
                      tunnel: w522 -> [w537] mode=indexing
                      tunnel: w520 -> [w534]
                      n237 = call-dynamic "Read Group.vi"("error in (no error)"=w536, "ObjectSettings in"=w537) -> ("error out"=w535:errorcluster, "Group"=w533:string, "ObjectSettings out"=w538:refnum<class "Path Settings.lvclass">)  [unwired: 7 in]
                      n238 = Equal?(x=w534, y=w533) -> (x = y?=w531:bool)
                      n239 = call-dynamic "Read GUID.vi"("error in (no error)"=w535, "ObjectSettings in"=w538) -> ("error out"=w541:errorcluster, "GUID"=w542:string, "ObjectSettings out"=w532:refnum<class "Path Settings.lvclass">)  [unwired: 7 in]
                      n240 = call-dynamic "Write GUID.vi"("error in (no error)"=w541, "GUID"=w542, "ObjectSettings in"=w539) -> ("error out"=w540:errorcluster, "ObjectSettings out"=w530:refnum<class "Path Settings.lvclass">)  [unwired: 7 in]
                      n241 = Select(t=w530, s=w531, f=w532) -> (s? t:f=w529:refnum<class "Path Settings.lvclass">)
                    }
                    n242 = call "Write Paths.vi"("error in (no error)"=w518, "Paths"=w523, "Setting Database in"=w525) -> ("error out"=w517:errorcluster, "Setting Database out"=w524:refnum<class "Setting Database.lvclass">)  [unwired: 7 in]
                  }
                  frame "r" {
                    n243 = call "Read Rectangles.vi"("error in (no error)"=w547, "Setting Database in"=w555) -> ("error out"=w549:errorcluster, "Rectangles"=w550:refnum<class "Rectangle Settings.lvclass">[], "Setting Database out"=w554:refnum<class "Setting Database.lvclass">)  [unwired: 7 in]
                    n244 = call "Read Active Rectangle.vi"("error in (no error)"=w549, "Setting Database in"=w554) -> ("error out"=w548:errorcluster, "Active Rectangle"=w551:refnum<class "Rectangle Settings.lvclass">, "Setting Database out"=w552:refnum<class "Setting Database.lvclass">)  [unwired: 7 in]
                    n245 = for {
                      shift-right: [w568] -> w545
                      shift-left: w548 -> [w564]
                      tunnel: [w557] -> w546 mode=indexing
                      tunnel: w551 -> [w567]
                      tunnel: w550 -> [w565] mode=indexing
                      tunnel: w556 -> [w562]
                      n246 = call-dynamic "Read Group.vi"("error in (no error)"=w564, "ObjectSettings in"=w565) -> ("error out"=w563:errorcluster, "Group"=w561:string, "ObjectSettings out"=w566:refnum<class "Rectangle Settings.lvclass">)  [unwired: 7 in]
                      n247 = Equal?(x=w562, y=w561) -> (x = y?=w559:bool)
                      n248 = call-dynamic "Read GUID.vi"("error in (no error)"=w563, "ObjectSettings in"=w566) -> ("error out"=w569:errorcluster, "GUID"=w570:string, "ObjectSettings out"=w560:refnum<class "Rectangle Settings.lvclass">)  [unwired: 7 in]
                      n249 = call-dynamic "Write GUID.vi"("error in (no error)"=w569, "GUID"=w570, "ObjectSettings in"=w567) -> ("error out"=w568:errorcluster, "ObjectSettings out"=w558:refnum<class "Rectangle Settings.lvclass">)  [unwired: 7 in]
                      n250 = Select(t=w558, s=w559, f=w560) -> (s? t:f=w557:refnum<class "Rectangle Settings.lvclass">)
                    }
                    n251 = call "Write Rectangles.vi"("error in (no error)"=w545, "Rectangles"=w546, "Setting Database in"=w552) -> ("error out"=w544:errorcluster, "Setting Database out"=w553:refnum<class "Setting Database.lvclass">)  [unwired: 7 in]
                  }
                  frame "f" {
                    n252 = call "Read Funnels.vi"("error in (no error)"=w579, "Setting Database in"=w580) -> ("error out"=w582:errorcluster, "Funnels"=w577:refnum<class "Funnel Settings.lvclass">[], "Setting Database out"=w581:refnum<class "Setting Database.lvclass">)  [unwired: 7 in]
                    n253 = call "Read Active Funnel.vi"("error in (no error)"=w582, "Setting Database in"=w581) -> ("error out"=w578:errorcluster, "Active Funnel"=w576:refnum<class "Funnel Settings.lvclass">, "Setting Database out"=w583:refnum<class "Setting Database.lvclass">)  [unwired: 7 in]
                    n254 = for {
                      shift-right: [w596] -> w574
                      shift-left: w578 -> [w592]
                      tunnel: [w585] -> w575 mode=indexing
                      tunnel: w576 -> [w595]
                      tunnel: w577 -> [w593] mode=indexing
                      tunnel: w584 -> [w590]
                      n255 = call-dynamic "Read Group.vi"("error in (no error)"=w592, "ObjectSettings in"=w593) -> ("error out"=w591:errorcluster, "Group"=w589:string, "ObjectSettings out"=w594:refnum<class "Funnel Settings.lvclass">)  [unwired: 7 in]
                      n256 = Equal?(x=w590, y=w589) -> (x = y?=w587:bool)
                      n257 = call-dynamic "Read GUID.vi"("error in (no error)"=w591, "ObjectSettings in"=w594) -> ("error out"=w597:errorcluster, "GUID"=w598:string, "ObjectSettings out"=w588:refnum<class "Funnel Settings.lvclass">)  [unwired: 7 in]
                      n258 = call-dynamic "Write GUID.vi"("error in (no error)"=w597, "GUID"=w598, "ObjectSettings in"=w595) -> ("error out"=w596:errorcluster, "ObjectSettings out"=w586:refnum<class "Funnel Settings.lvclass">)  [unwired: 7 in]
                      n259 = Select(t=w586, s=w587, f=w588) -> (s? t:f=w585:refnum<class "Funnel Settings.lvclass">)
                    }
                    n260 = call "Write Funnels.vi"("error in (no error)"=w574, "Funnels"=w575, "Setting Database in"=w583) -> ("error out"=w573:errorcluster, "Setting Database out"=w572:refnum<class "Setting Database.lvclass">)  [unwired: 7 in]
                  }
                  frame "d" {
                    n261 = call "Read Dots.vi"("error in (no error)"=w608, "Setting Database in"=w611) -> ("error out"=w607:errorcluster, "Dots"=w610:refnum<class "Dot Settings.lvclass">[], "Setting Database out"=w609:refnum<class "Setting Database.lvclass">)  [unwired: 7 in]
                    n262 = call "Read Active Dot.vi"("error in (no error)"=w607, "Setting Database in"=w609) -> ("error out"=w606:errorcluster, "Active Dot"=w605:refnum<class "Dot Settings.lvclass">, "Setting Database out"=w603:refnum<class "Setting Database.lvclass">)  [unwired: 7 in]
                    n263 = for {
                      shift-right: [w624] -> w601
                      shift-left: w606 -> [w620]
                      tunnel: [w613] -> w602 mode=indexing
                      tunnel: w605 -> [w623]
                      tunnel: w610 -> [w621] mode=indexing
                      tunnel: w612 -> [w618]
                      n264 = call-dynamic "Read Group.vi"("error in (no error)"=w620, "ObjectSettings in"=w621) -> ("error out"=w619:errorcluster, "Group"=w617:string, "ObjectSettings out"=w622:refnum<class "Dot Settings.lvclass">)  [unwired: 7 in]
                      n265 = Equal?(x=w618, y=w617) -> (x = y?=w615:bool)
                      n266 = call-dynamic "Read GUID.vi"("error in (no error)"=w619, "ObjectSettings in"=w622) -> ("error out"=w625:errorcluster, "GUID"=w626:string, "ObjectSettings out"=w616:refnum<class "Dot Settings.lvclass">)  [unwired: 7 in]
                      n267 = call-dynamic "Write GUID.vi"("error in (no error)"=w625, "GUID"=w626, "ObjectSettings in"=w623) -> ("error out"=w624:errorcluster, "ObjectSettings out"=w614:refnum<class "Dot Settings.lvclass">)  [unwired: 7 in]
                      n268 = Select(t=w614, s=w615, f=w616) -> (s? t:f=w613:refnum<class "Dot Settings.lvclass">)
                    }
                    n269 = call "Write Dots.vi"("error in (no error)"=w601, "Dots"=w602, "Setting Database in"=w603) -> ("error out"=w600:errorcluster, "Setting Database out"=w604:refnum<class "Setting Database.lvclass">)  [unwired: 7 in]
                  }
                }
                n270 = Bundle By Name(cluster=w505, "Self"=w504) -> (w506:T6)
                n271 = call <vilib>:"Add State(s) to Queue__jki_lib_state_machine.vi"("State(s) in Front (\"\")"=w500, "State(s) in (\"\")"=w509) -> ("States Out"=w508:string)  [unwired: 13 in]
              }
              event User Event {
                n272 = event-data() -> ()  [unwired: 1 in, 5 out]
                n273 = Unbundle By Name(w640) -> ("Self"=w638:refnum<class "Setting Database.lvclass">)
                n274 = call "Read Dots.vi"("error in (no error)"=w633, "Setting Database in"=w638) -> ("error out"=w634:errorcluster, "Dots"=w630:refnum<class "Dot Settings.lvclass">[], "Setting Database out"=w636:refnum<class "Setting Database.lvclass">)  [unwired: 7 in]
                n275 = call "Read Active Dot.vi"("error in (no error)"=w634, "Setting Database in"=w636) -> ("error out"=w628:errorcluster, "Active Dot"=w631:refnum<class "Dot Settings.lvclass">, "Setting Database out"=w635:refnum<class "Setting Database.lvclass">)  [unwired: 7 in]
                n276 = for {
                  shift-right: [w646] -> w627
                  shift-left: w628 -> [w648]
                  tunnel: [w647] -> w629 mode=indexing
                  tunnel: w631 -> [w645]
                  tunnel: w630 -> [w644] mode=indexing
                  n277 = call-dynamic "Read GUID.vi"("error in (no error)"=w648, "ObjectSettings in"=w644) -> ("error out"=w649:errorcluster, "GUID"=w650:string)  [unwired: 7 in, 1 out]
                  n278 = call-dynamic "Write GUID.vi"("error in (no error)"=w649, "GUID"=w650, "ObjectSettings in"=w645) -> ("error out"=w646:errorcluster, "ObjectSettings out"=w647:refnum<class "Dot Settings.lvclass">)  [unwired: 7 in]
                }
                n279 = call "Write Dots.vi"("error in (no error)"=w627, "Dots"=w629, "Setting Database in"=w635) -> ("error out"=w632:errorcluster, "Setting Database out"=w637:refnum<class "Setting Database.lvclass">)  [unwired: 7 in]
                n280 = Bundle By Name(cluster=w640, "Self"=w637) -> (w641:T6)
                n281 = call <vilib>:"Add State(s) to Queue__jki_lib_state_machine.vi"("State(s) in Front (\"\")"="Publish: Dots", "State(s) in (\"\")"=w643) -> ("States Out"=w642:string)  [unwired: 13 in]
              }
              event User Event {
                n282 = event-data() -> ()  [unwired: 1 in, 1 out]
                n283 = Unbundle By Name(w664) -> ("Self"=w663:refnum<class "Setting Database.lvclass">)
                n284 = call "Read Rectangles.vi"("error in (no error)"=w662, "Setting Database in"=w663) -> ("error out"=w660:errorcluster, "Rectangles"=w653:refnum<class "Rectangle Settings.lvclass">[], "Setting Database out"=w661:refnum<class "Setting Database.lvclass">)  [unwired: 7 in]
                n285 = call "Read Active Rectangle.vi"("error in (no error)"=w660, "Setting Database in"=w661) -> ("error out"=w652:errorcluster, "Active Rectangle"=w655:refnum<class "Rectangle Settings.lvclass">, "Setting Database out"=w659:refnum<class "Setting Database.lvclass">)  [unwired: 7 in]
                n286 = for {
                  tunnel: w653 -> [w674] mode=indexing
                  tunnel: w655 -> [w673]
                  shift-right: [w668] -> w651
                  shift-left: w652 -> [w670]
                  tunnel: [w669] -> w654 mode=indexing
                  n287 = call-dynamic "Read GUID.vi"("error in (no error)"=w670, "ObjectSettings in"=w674) -> ("error out"=w671:errorcluster, "GUID"=w672:string)  [unwired: 7 in, 1 out]
                  n288 = call-dynamic "Write GUID.vi"("error in (no error)"=w671, "GUID"=w672, "ObjectSettings in"=w673) -> ("error out"=w668:errorcluster, "ObjectSettings out"=w669:refnum<class "Rectangle Settings.lvclass">)  [unwired: 7 in]
                }
                n289 = call "Write Rectangles.vi"("error in (no error)"=w651, "Rectangles"=w654, "Setting Database in"=w659) -> ("error out"=w657:errorcluster, "Setting Database out"=w658:refnum<class "Setting Database.lvclass">)  [unwired: 7 in]
                n290 = Bundle By Name(cluster=w664, "Self"=w658) -> (w665:T6)
                n291 = call <vilib>:"Add State(s) to Queue__jki_lib_state_machine.vi"("State(s) in Front (\"\")"="Publish: Rectangles", "State(s) in (\"\")"=w667) -> ("States Out"=w666:string)  [unwired: 13 in]
              }
              event User Event {
                n292 = event-data() -> ()  [unwired: 1 in, 1 out]
                n293 = Unbundle By Name(w688) -> ("Self"=w686:refnum<class "Setting Database.lvclass">)
                n294 = call "Read Funnels.vi"("error in (no error)"=w675, "Setting Database in"=w686) -> ("error out"=w684:errorcluster, "Funnels"=w680:refnum<class "Funnel Settings.lvclass">[], "Setting Database out"=w685:refnum<class "Setting Database.lvclass">)  [unwired: 7 in]
                n295 = call "Read Active Funnel.vi"("error in (no error)"=w684, "Setting Database in"=w685) -> ("error out"=w676:errorcluster, "Active Funnel"=w677:refnum<class "Funnel Settings.lvclass">, "Setting Database out"=w682:refnum<class "Setting Database.lvclass">)  [unwired: 7 in]
                n296 = for {
                  tunnel: w680 -> [w698] mode=indexing
                  tunnel: w677 -> [w697]
                  shift-right: [w692] -> w679
                  shift-left: w676 -> [w694]
                  tunnel: [w693] -> w678 mode=indexing
                  n297 = call-dynamic "Read GUID.vi"("error in (no error)"=w694, "ObjectSettings in"=w698) -> ("error out"=w695:errorcluster, "GUID"=w696:string)  [unwired: 7 in, 1 out]
                  n298 = call-dynamic "Write GUID.vi"("error in (no error)"=w695, "GUID"=w696, "ObjectSettings in"=w697) -> ("error out"=w692:errorcluster, "ObjectSettings out"=w693:refnum<class "Funnel Settings.lvclass">)  [unwired: 7 in]
                }
                n299 = call "Write Funnels.vi"("error in (no error)"=w679, "Funnels"=w678, "Setting Database in"=w682) -> ("error out"=w681:errorcluster, "Setting Database out"=w683:refnum<class "Setting Database.lvclass">)  [unwired: 7 in]
                n300 = Bundle By Name(cluster=w688, "Self"=w683) -> (w689:T6)
                n301 = call <vilib>:"Add State(s) to Queue__jki_lib_state_machine.vi"("State(s) in Front (\"\")"="Publish: Funnels", "State(s) in (\"\")"=w691) -> ("States Out"=w690:string)  [unwired: 13 in]
              }
              event User Event {
                n302 = event-data() -> ("SetCurrentPath"=w700:T9)  [unwired: 1 in]
                n303 = Unbundle By Name(w708) -> ("Self"=w706:refnum<class "Setting Database.lvclass">)
                n304 = call "Read Active.vi"("error in (no error)"=w712, "Setting Database in"=w706) -> ("error out"=w699:errorcluster, "Active"=w704:T10, "Setting Database out"=w705:refnum<class "Setting Database.lvclass">)  [unwired: 7 in]
                n305 = Bundle By Name(cluster=w704, "Path"=w700) -> (w703:T10)
                n306 = call "Write Active.vi"("error in (no error)"=w699, "Active"=w703, "Setting Database in"=w705) -> ("error out"=w701:errorcluster, "Setting Database out"=w702:refnum<class "Setting Database.lvclass">)  [unwired: 7 in]
                n307 = Bundle By Name(cluster=w708, "Self"=w702) -> (w709:T6)
                n308 = call <vilib>:"Add State(s) to Queue__jki_lib_state_machine.vi"("State(s) in Front (\"\")"="Publish: Active Path" ("State(s) in Front (\"\")"), "State(s) in (\"\")"=w711) -> ("States Out"=w710:string)  [unwired: 13 in]
              }
              event User Event {
                n309 = event-data() -> ("SetActiveDot"=w714:T11)  [unwired: 1 in]
                n310 = Unbundle By Name(w720) -> ("Self"=w717:refnum<class "Setting Database.lvclass">)
                n311 = call "Read Active.vi"("error in (no error)"=w724, "Setting Database in"=w717) -> ("error out"=w726:errorcluster, "Active"=w715:T10, "Setting Database out"=w716:refnum<class "Setting Database.lvclass">)  [unwired: 7 in]
                n312 = Bundle By Name(cluster=w715, "Dot"=w714) -> (w713:T10)
                n313 = call "Write Active.vi"("error in (no error)"=w726, "Active"=w713, "Setting Database in"=w716) -> ("error out"=w725:errorcluster, "Setting Database out"=w719:refnum<class "Setting Database.lvclass">)  [unwired: 7 in]
                n314 = Bundle By Name(cluster=w720, "Self"=w719) -> (w721:T6)
                n315 = call <vilib>:"Add State(s) to Queue__jki_lib_state_machine.vi"("State(s) in Front (\"\")"="Publish: Active Dot" ("State(s) in Front (\"\")"), "State(s) in (\"\")"=w723) -> ("States Out"=w722:string)  [unwired: 13 in]
              }
              event User Event {
                n316 = event-data() -> ("SetActiveRectangle"=w728:T12)  [unwired: 1 in]
                n317 = Unbundle By Name(w734) -> ("Self"=w731:refnum<class "Setting Database.lvclass">)
                n318 = call "Read Active.vi"("error in (no error)"=w738, "Setting Database in"=w731) -> ("error out"=w740:errorcluster, "Active"=w729:T10, "Setting Database out"=w730:refnum<class "Setting Database.lvclass">)  [unwired: 7 in]
                n319 = Bundle By Name(cluster=w729, "Rectangle"=w728) -> (w727:T10)
                n320 = call "Write Active.vi"("error in (no error)"=w740, "Active"=w727, "Setting Database in"=w730) -> ("error out"=w739:errorcluster, "Setting Database out"=w733:refnum<class "Setting Database.lvclass">)  [unwired: 7 in]
                n321 = Bundle By Name(cluster=w734, "Self"=w733) -> (w735:T6)
                n322 = call <vilib>:"Add State(s) to Queue__jki_lib_state_machine.vi"("State(s) in Front (\"\")"="Publish: Active Rectangle" ("State(s) in Front (\"\")"), "State(s) in (\"\")"=w737) -> ("States Out"=w736:string)  [unwired: 13 in]
              }
              event User Event {
                n323 = event-data() -> ("SetActiveFunnel"=w742:T13)  [unwired: 1 in]
                n324 = Unbundle By Name(w748) -> ("Self"=w745:refnum<class "Setting Database.lvclass">)
                n325 = call "Read Active.vi"("error in (no error)"=w752, "Setting Database in"=w745) -> ("error out"=w754:errorcluster, "Active"=w743:T10, "Setting Database out"=w744:refnum<class "Setting Database.lvclass">)  [unwired: 7 in]
                n326 = Bundle By Name(cluster=w743, "Funnel"=w742) -> (w741:T10)
                n327 = call "Write Active.vi"("error in (no error)"=w754, "Active"=w741, "Setting Database in"=w744) -> ("error out"=w753:errorcluster, "Setting Database out"=w747:refnum<class "Setting Database.lvclass">)  [unwired: 7 in]
                n328 = Bundle By Name(cluster=w748, "Self"=w747) -> (w749:T6)
                n329 = call <vilib>:"Add State(s) to Queue__jki_lib_state_machine.vi"("State(s) in Front (\"\")"="Publish: Active Funnel" ("State(s) in Front (\"\")"), "State(s) in (\"\")"=w751) -> ("States Out"=w750:string)  [unwired: 13 in]
              }
              event User Event {
                n330 = event-data() -> ("UpdateCurrentPath"=w758:T14)  [unwired: 1 in]
                n331 = Unbundle By Name(w761) -> ("Self"=w760:refnum<class "Setting Database.lvclass">)
                n332 = call "Write Active Path.vi"("error in (no error)"=w755, "Path Settings.lvclass"=w758, "Setting Database in"=w760) -> ("error out"=w756:errorcluster, "Setting Database out"=w759:refnum<class "Setting Database.lvclass">)  [unwired: 7 in]
                n333 = Bundle By Name(cluster=w761, "Self"=w759) -> (w762:T6)
                n334 = call <vilib>:"Add State(s) to Queue__jki_lib_state_machine.vi"("State(s) in Front (\"\")"="Publish: Paths", "State(s) in (\"\")"=w764) -> ("States Out"=w763:string)  [unwired: 13 in]
              }
              event User Event {
                # "We publish the active here as well because we have a subsub panel thing going on (dots edit and then IV curve and Quantum Dot situation) and it is basically to make sure that if we update the sub panel it will also change the information in the sub sub panel and vice versa"
                n335 = event-data() -> ("UpdateActiveDot"=w765:T15)  [unwired: 1 in]
                n336 = Unbundle By Name(w771) -> ("Self"=w769:refnum<class "Setting Database.lvclass">)
                n337 = call "Write Active Dot.vi"("error in (no error)"=w767, "Active Dot"=w765, "Setting Database in"=w769) -> ("error out"=w766:errorcluster, "Setting Database out"=w768:refnum<class "Setting Database.lvclass">)  [unwired: 7 in]
                n338 = Bundle By Name(cluster=w771, "Self"=w768) -> (w772:T6)
                n339 = call <vilib>:"Add State(s) to Queue__jki_lib_state_machine.vi"("State(s) in Front (\"\")"="Publish: Active Dot\nPublish: Dots", "State(s) in (\"\")"=w774) -> ("States Out"=w773:string)  [unwired: 13 in]
              }
              event User Event {
                n340 = event-data() -> ("UpdateActiveRectangle"=w775:T16)  [unwired: 1 in]
                n341 = Unbundle By Name(w781) -> ("Self"=w779:refnum<class "Setting Database.lvclass">)
                n342 = call "Write Active Rectangle.vi"("error in (no error)"=w777, "Active Rectangle"=w775, "Setting Database in"=w779) -> ("error out"=w776:errorcluster, "Setting Database out"=w778:refnum<class "Setting Database.lvclass">)  [unwired: 7 in]
                n343 = Bundle By Name(cluster=w781, "Self"=w778) -> (w782:T6)
                n344 = call <vilib>:"Add State(s) to Queue__jki_lib_state_machine.vi"("State(s) in Front (\"\")"="Publish: Rectangles", "State(s) in (\"\")"=w784) -> ("States Out"=w783:string)  [unwired: 13 in]
              }
              event User Event {
                n345 = event-data() -> ("UpdateActiveFunnel"=w785:T17)  [unwired: 1 in]
                n346 = Unbundle By Name(w791) -> ("Self"=w789:refnum<class "Setting Database.lvclass">)
                n347 = call "Write Active Funnel.vi"("error in (no error)"=w787, "Active Funnel"=w785, "Setting Database in"=w789) -> ("error out"=w786:errorcluster, "Setting Database out"=w788:refnum<class "Setting Database.lvclass">)  [unwired: 7 in]
                n348 = Bundle By Name(cluster=w791, "Self"=w788) -> (w792:T6)
                n349 = call <vilib>:"Add State(s) to Queue__jki_lib_state_machine.vi"("State(s) in Front (\"\")"="Publish: Funnels", "State(s) in (\"\")"=w794) -> ("States Out"=w793:string)  [unwired: 13 in]
              }
              event Panel Close? {
                # "Discard the event because we'll close the front panel ourselves in Macro: Exit"
                # "Close Panel button (pressed) Event\n(this executes Macro: Exit to terminate the VI)"
                n350 = event-data() -> ()  [unwired: 1 in, 1 out]
                n351 = event-data("Discard?"=FALSE) -> ()  [unwired: 1 in, 1 out]
                n352 = call <vilib>:"Add State(s) to Queue__jki_lib_state_machine.vi"("State(s) in Front (\"\")"="//Macro: Exit", "State(s) in (\"\")"=w799) -> ("States Out"=w798:string)  [unwired: 13 in]
              }
              event User Event {
                n353 = event-data() -> ()  [unwired: 1 in, 5 out]
                n354 = call <vilib>:"Add State(s) to Queue__jki_lib_state_machine.vi"("State(s) in Front (\"\")"="Macro: Exit", "State(s) in (\"\")"=w804) -> ("States Out"=w803:string)  [unwired: 13 in]
              }
              event User Event {
                # "On Abort, no nice macro exit, but exit right away"
                n355 = event-data() -> ()  [unwired: 1 in, 5 out]
                n356 = call <vilib>:"Add State(s) to Queue__jki_lib_state_machine.vi"("State(s) in Front (\"\")"="Exit", "State(s) in (\"\")"=w809) -> ("States Out"=w808:string)  [unwired: 13 in]
              }
            }
          }
          frame "---------- Core ----------" {
            # "Do not put any code in this frame.\n(it is a separator no-op)"
            n357 = call <vilib>:"Add State(s) to Queue__jki_lib_state_machine.vi"("State(s) in (\"\")"=w814) -> ("States Out"=w813:string)  [unwired: 14 in]
          }
          frame Default {
            w823 = 42 items=["No error", "Argument error", "Memory is full", "Out of zone", "End of file", "File already open", "Generic file I/O error", "File not found", "File permission error", "Disk is full", "Duplicate path", "Too many files open", "System feature not enabled", "Resource file not found", "Cannot add resource", "Resource not found", "Image not found", "Image memory error", "Pen does not exist", "Config type invalid", "Config token not found", "Config parse error", "Config memory error", "Bad external code format", "Bad external code offset", "External code not present", "Null window", "Destroy window error", "Null menu", "Print aborted", "Bad print record", "Print driver error", "Windows error during printing", "Memory error during printing", "Print dialog error", "Generic print error", "Invalid device refnum", "Device not found", "Device parameter error", "Device unit error", "Cannot open device", "Device call aborted", "Generic error", "Cancelled by user", "Object ID too low", "Object ID too high", "Object not in heap", "Unknown heap", "Unknown object (invalid DefProc)", "Unknown object (DefProc not in table)", "Message out of range", "Invalid (null) method", "Unknown message", "Manager call not supported", "Bad address", "Network operation in progress", "Network operation timed out", "Connection is busy", "Network attribute not supported", "Network error", "Address in use", "System out of memory", "Connection aborted", "Connection refused", "Not connected", "Already connected", "Connection closed", "Initialization error (interapplication manager)", "Bad occurrence", "Wait on unbound occurrence handler", "Occurrence queue overflow", "Datalog type conflict", "Unused", "Unrecognized type (interapplication manager)", "Memory corrupt", "Failed to make temporary DLL", "Old CIN version", "Drag socket not found", "Failed to load drop-object", "Failed to register OLE object", "Failed to release OLE object", "Format specifier type mismatch", "Unknown format specifier", "Too few format specifiers", "Too many format specifiers", "Scan failed", "Newer CIN version", "Error converting to variant", "Runtime menu error", "Password tampered", "Variant attribute not found", "Incompatible variant data type", "Event data is not available", "Event Store is not present", "Occurrence is not found", "Event Queue is not created", "Event info is not available", "Refnum passed is NULL", "Error retrieving Class GUID", "Error retrieving CoClass GUID", "Error retrieving TypeLib GUID.", "Bad built application magic bytes.", "Specific driver is different from the specific driver associated with the Logical Name.", "There is no session opened to the class driver.", "Max Error", "MAX - Error with config objects", "MAX - Error loading configuration", "MAX - Group not supported"]
            # "Current State"
            # "Do not delete, rename, or modify this frame.\n(this is used to capture unhandled states and typos)"
            # "Handle mistyped state name (developer tool)"
            n358 = Format Into String(format string="Software Exception: Unhandled State \"%s\"." ("message"), error in=w825, w817) -> (resulting string=w822:string, error out=w827:errorcluster)  [unwired: 1 in]
            n359 = call <vilib>:"Error Cluster From Error Code.vi"("show call chain? (False)"=TRUE, "error in (no error)"=w827, "error message (\"\")"=w822, "error code (0)"=w823) -> ("error out"=w826:errorcluster)  [unwired: 5 in]
            n360 = call <vilib>:"Add State(s) to Queue__jki_lib_state_machine.vi"("State(s) in (\"\")"=w821) -> ("States Out"=w820:string)  [unwired: 14 in]
          }
          frame "Initialize Core Data" {
            # "Do not delete, rename, or modify this frame.\n(this is used to determine panel behavior on exit)"
            # "originally closed?"
            # "exe?"
            # "If panel starts closed or is an EXE, then close it when we exit"
            n361 = property class="VI"() -> ("Front Panel.Open"=w836:bool)  [unwired: 2 in, 2 out]
            n362 = property class="App"() -> ("App.Kind"=w835:T3)  [unwired: 2 in, 2 out]
            n363 = control-ref of="Current VI Reference"() -> (w829:refnum<vi>)
            n364 = Not(x=w836) -> (.not. x?=w833:bool)
            n365 = Equal?(x=w835, y=T3."Run Time System" ("Application:Kind")) -> (x = y?=w832:bool)
            n366 = Or(x=w833, y=w832) -> (x .or. y?=w830:bool)
            n367 = Bundle By Name(cluster=w831, "Core.Current VI Reference"=w829, "Core.Close Panel on Exit?"=w830) -> (w837:T6)
            n368 = call <vilib>:"Add State(s) to Queue__jki_lib_state_machine.vi"("State(s) in (\"\")"=w839) -> ("States Out"=w838:string)  [unwired: 14 in]
          }
          frame "Error Handler" {
            w841 = TRUE  # Stop on Unhandled Error (T)
            w853 = errorcluster {"status"=FALSE, "code"=0, "source"=""}  # No error
            # "Overwrite this method to handle errors and pass to parent if not handled. Parent will fire a public event if the error is not handled up the chain of classes."
            n369 = Unbundle By Name(w846) -> ("Self"=w847:refnum<class "Setting Database.lvclass">)
            n370 = call-dynamic "Handle Error.vi"("Stop on Unhandled Error (T)"=w841, "error in"=w854, "SMO"=w847) -> ("handling error"=w851:errorcluster, "Unhandled error"=w852:errorcluster)  [unwired: 6 in, 1 out]
            n371 = Bundle By Name(cluster=w846, "Core.error"=w852) -> (w845:T6)
            n372 = Select(t="Exit", s=w851, f="") -> (s? t:f=w844:string)
            n373 = call <vilib>:"Add State(s) to Queue__jki_lib_state_machine.vi"("State(s) in Front (\"\")"=w844, "State(s) in (\"\")"=w850) -> ("States Out"=w849:string)  [unwired: 13 in]
          }
          frame "Exit" {
            # "Do not put any code in this frame.\n(No errors that occur here will be handled.)"
            n374 = Unbundle By Name(w855) -> ("Core.error"=w860:errorcluster)
            n375 = call <vilib>:"Add State(s) to Queue__jki_lib_state_machine.vi"("State(s) in (\"\")"=w859) -> ("States Out"=w858:string)  [unwired: 14 in]
          }
          frame "---------- Data ----------" {
            # "Do not put any code in this frame.\n(It is a separator no-op. You can make a copy of this frame to create a new Data frame)"
            n376 = call <vilib>:"Add State(s) to Queue__jki_lib_state_machine.vi"("State(s) in (\"\")"=w864) -> ("States Out"=w863:string)  [unwired: 14 in]
          }
          frame "Data: Read Defaults" {
            # "Do not put any code in this frame.\n(It is a separator no-op. You can make a copy of this frame to create a new Data frame)"
            n377 = Unbundle By Name(w871) -> ("Self"=w867:refnum<class "Setting Database.lvclass">)
            n378 = call "Base INI Folder Path.vi"() -> ("Base Path"=w866:path)  [unwired: 11 in]
            n379 = call "RetrieveDefaultDotData.vi"("error in (no error)"=w868, "Path"=w866, "Setting Database In"=w867) -> ("error out"=w877:errorcluster, "Setting Database Out"=w878:refnum<class "Setting Database.lvclass">)  [unwired: 6 in, 1 out]
            n380 = call "RetrieveDefaultPathData.vi"("error in (no error)"=w877, "Path"=w866, "Setting Database In"=w878) -> ("error out"=w875:errorcluster, "Setting Database Out"=w876:refnum<class "Setting Database.lvclass">)  [unwired: 6 in, 1 out]
            n381 = call "RetrieveDefaultFunnelData.vi"("error in (no error)"=w875, "Path"=w866, "Setting Database In"=w876) -> ("error out"=w873:errorcluster, "Setting Database Out"=w874:refnum<class "Setting Database.lvclass">)  [unwired: 6 in, 1 out]
            n382 = call "RetrieveDefaultRectangleData.vi"("error in (no error)"=w873, "Path"=w866, "Setting Database In"=w874) -> ("error out"=w870:errorcluster, "Setting Database Out"=w869:refnum<class "Setting Database.lvclass">)  [unwired: 6 in, 1 out]
            n383 = Bundle By Name(cluster=w871, "Self"=w869) -> (w872:T6)
            n384 = call <vilib>:"Add State(s) to Queue__jki_lib_state_machine.vi"("State(s) in (\"\")"=w881) -> ("States Out"=w880:string)  [unwired: 14 in]
          }
          frame "Data: Initialize" {
            w882 = refnum<class "Setting Database.lvclass"> refnum  # Self
            w885 = T18 {"Current VI Reference"=refnum, "Close Panel on Exit?"=FALSE, "error"={"status"=FALSE, "code"=0, "source"=""}}  # Core
            # "do not delete - used by framework"
            # "Expand Bundle to add new data elements to shift register data."
            # "Add new data here."
            # "Data names and types of shift register data are defined by this bundle."
            # "Initialize the shift-register data, here.\n(data names are defined by what you wire into the bundle function)"
            n385 = Variant To Data(error in=w891, type=w882, Variant=w887) -> (data=w884:refnum<class "Setting Database.lvclass">, error out=w890:errorcluster)
            n386 = Bundle("Core"=w885, "Self"=w884) -> (w883:T6)  [unwired: 1 in]
            n387 = call <vilib>:"Add State(s) to Queue__jki_lib_state_machine.vi"("State(s) in (\"\")"=w889) -> ("States Out"=w888:string)  [unwired: 14 in]
          }
          frame "Data: Cleanup" {
            # "Cleanup any data and references, here.\n(this is called automatically, by the Macro: Exit)"
            n388 = Unbundle By Name(w893) -> ("Core.Current VI Reference"=w894:refnum<vi>)
            n389 = Close Reference(reference=w894, error in (no error)=w898) -> (error out=w897:errorcluster)
            n390 = call <vilib>:"Add State(s) to Queue__jki_lib_state_machine.vi"("State(s) in (\"\")"=w896) -> ("States Out"=w895:string)  [unwired: 14 in]
          }
          frame "---------- UI ----------" {
            # "Do not put any code in this frame.\n(It is a separator no-op. You can make a copy of this frame to create a new UI frame)"
            n391 = call <vilib>:"Add State(s) to Queue__jki_lib_state_machine.vi"("State(s) in (\"\")"=w902) -> ("States Out"=w901:string)  [unwired: 14 in]
          }
          frame "UI: Initialize" {
            # "Initialize the User Interface, here.\n(this is called automatically, by the Macro: Init)"
            n392 = call <vilib>:"Add State(s) to Queue__jki_lib_state_machine.vi"("State(s) in (\"\")"=w907) -> ("States Out"=w906:string)  [unwired: 14 in]
          }
          frame "UI: Cursor Set" {
            # "Argument"
            # "Initialize the User Interface, here.\n(this is called automatically, by the Macro: Init)"
            n393 = disable-structure shown="Default" {
              disable-tunnel: w915 -> [w916 w919]
              disable-tunnel: [w916 w918] -> w914
              disable-tunnel: w909 -> [_ w917]
              frame condition #0 {
              }
              frame condition #1 (active) {
                n394 = case shown="\"Idle\", Default" w917 {
                  tunnel: w919 -> [w921 w923]
                  tunnel: [w920 w922] -> w918
                  frame "Idle", Default {
                    n395 = call <vilib>:"Unset Busy.vi"("error in (no error)"=w921) -> ("error out"=w920:errorcluster)  [unwired: 10 in]
                  }
                  frame "Busy" {
                    n396 = call <vilib>:"Set Busy.vi"("error in (no error)"=w923) -> ("error out"=w922:errorcluster)  [unwired: 9 in, 1 out]
                  }
                }
              }
            }
            n397 = call <vilib>:"Add State(s) to Queue__jki_lib_state_machine.vi"("State(s) in (\"\")"=w913) -> ("States Out"=w912:string)  [unwired: 14 in]
          }
          frame "UI: Front Panel State" {
            # "Argument"
            # "Set Front Panel Open or Closed\n(Usage: \"UI: Front Panel State >> Open|Close\")"
            n398 = Unbundle By Name(w927) -> ("Core.Current VI Reference"=w926:refnum<vi>)
            n399 = disable-structure shown="Default" {
              disable-tunnel: w931 -> [w935 w958]
              disable-tunnel: [w934 w958] -> w930
              disable-tunnel: w926 -> [w933 _]
              disable-tunnel: w925 -> [w932 _]
              frame condition #0 (active) {
                n400 = case shown="\"Close\"" w932 {
                  tunnel: w935 -> [w940 w952]
                  tunnel: [w941 w953] -> w934
                  tunnel: w933 -> [w938 w950]
                  frame "Open", Default {
                    n401 = property class="VI"(reference=w938, error in=w940) -> (reference out=w937:refnum<vi>, error out=w939:errorcluster, "FP.State"=w936:T4)
                    n402 = case shown="\"Closed\"" w936 {
                      tunnel: [w946 w947] -> w941
                      tunnel: w939 -> [w945 w947]
                      tunnel: w937 -> [w942 _]
                      frame "Closed" {
                        n403 = invoke class="VI" method="FP.Open"(reference=w942, error in=w945, "Activate"=TRUE, "State"=T4."Standard") -> (error out=w946:errorcluster)  [unwired: 1 in, 4 out]
                      }
                      frame Default {
                      }
                    }
                  }
                  frame "Close" {
                    n404 = property class="VI"(reference=w950, error in=w952) -> (reference out=w949:refnum<vi>, error out=w951:errorcluster, "FP.State"=w948:T4)
                    n405 = case shown="Default" w948 {
                      tunnel: [w954 w957] -> w953
                      tunnel: w951 -> [w954 w956]
                      tunnel: w949 -> [_ w955]
                      frame "Invalid", "Closed" {
                      }
                      frame Default {
                        n406 = invoke class="VI" method="FP.Close"(reference=w955, error in=w956) -> (error out=w957:errorcluster)  [unwired: 1 in, 2 out]
                      }
                    }
                  }
                }
              }
              frame condition #1 {
              }
            }
            n407 = call <vilib>:"Add State(s) to Queue__jki_lib_state_machine.vi"("State(s) in (\"\")"=w929) -> ("States Out"=w928:string)  [unwired: 14 in]
          }
          frame "---------- Macro ----------" {
            # "Do not put any code in this frame.\n(It is a separator no-op. You can make a copy of this frame to create a new Macro frame)"
            n408 = call <vilib>:"Add State(s) to Queue__jki_lib_state_machine.vi"("State(s) in (\"\")"=w962) -> ("States Out"=w961:string)  [unwired: 14 in]
          }
          frame "Macro: Initialize" {
            w968 = "Data: Read Defaults\n//UI: Initialize\n//UI: Front Panel State >> Open"  # Data: Read Defaults //UI: Initialize //UI: Front Panel State >> Open
            w964 = "Process: Sync"
            # "Initialization Macro\n(This is called once, when the VI starts)"
            n409 = control-ref of="This VI"() -> (w966:refnum<vi>)
            n410 = property class="VI"(reference=w966) -> ("Exec.State"=w965:T5)  [unwired: 1 in, 2 out]
            n411 = Equal?(x=w965, y=T5."Run top level") -> (x = y?=w971:bool)
            n412 = Select(t=w964, s=w971, f="") -> ()  [unwired: 1 out]
            n413 = call <vilib>:"Add State(s) to Queue__jki_lib_state_machine.vi"("State(s) in Front (\"\")"="Data: Initialize\nInitialize Core Data\nEvents: Register", "State(s) in (\"\")"=w964, "State(s) at Back (\"\")"=w968) -> ("States Out"=w967:string)  [unwired: 12 in]
            n414 = call <vilib>:"Add State(s) to Queue__jki_lib_state_machine.vi"("State(s) in Front (\"\")"=w967, "State(s) in (\"\")"=w976) -> ("States Out"=w975:string)  [unwired: 13 in]
          }
          frame "Macro: Exit" {
            # "Exit Macro\n(This is called once, when the VI exits)"
            n415 = Unbundle By Name(w982) -> ("Core.Close Panel on Exit?"=w988:bool)
            n416 = Select(t="UI: Front Panel State >> Close", s=w988, f="") -> (s? t:f=w985:string)
            n417 = call <vilib>:"Add State(s) to Queue__jki_lib_state_machine.vi"("State(s) in Front (\"\")"="Data: Cleanup\nEvents: Unregister", "State(s) in (\"\")"="Process: Sync", "State(s) at Back (\"\")"="Exit") -> ("States Out"=w979:string)  [unwired: 12 in]
            n418 = call <vilib>:"Add State(s) to Queue__jki_lib_state_machine.vi"("State(s) in (\"\")"=w985, "State(s) at Back (\"\")"=w979) -> ("States Out"=w984:string)  [unwired: 13 in]
            n419 = call <vilib>:"Add State(s) to Queue__jki_lib_state_machine.vi"("State(s) in Front (\"\")"=w984, "State(s) in (\"\")"=w990) -> ("States Out"=w989:string)  [unwired: 13 in]
          }
          frame "---------- Process ----------" {
            # "Template Separator\n(You can make a copy of, or modify, this frame)"
            n420 = call <vilib>:"Add State(s) to Queue__jki_lib_state_machine.vi"("State(s) in (\"\")"=w995) -> ("States Out"=w994:string)  [unwired: 14 in]
          }
          frame "Process: Sync" {
            n421 = Unbundle By Name(w1002) -> ("Self"=w998:refnum<class "Setting Database.lvclass">)
            n422 = call <vilib>:"WaitOnProcessSync.vi"("error in (no error)"=w1007, "SMO"=w998) -> ("error out"=w1006:errorcluster, "Don't run?"=w1001:bool)  [unwired: 7 in, 1 out]
            n423 = Select(t="Data: Cleanup\nEvents: Unregister\nExit", s=w1001, f="") -> (s? t:f=w997:string)
            n424 = call <vilib>:"Add State(s) to Queue__jki_lib_state_machine.vi"("State(s) in Front (\"\")"=w997, "State(s) in (\"\")"=w1005) -> ("States Out"=w1004:string)  [unwired: 13 in]
          }
          frame "---------- Events ----------" {
            # "Template Separator\n(You can make a copy of, or modify, this frame)"
            n425 = call <vilib>:"Add State(s) to Queue__jki_lib_state_machine.vi"("State(s) in (\"\")"=w1011) -> ("States Out"=w1010:string)  [unwired: 14 in]
          }
          frame "Events: Register" {
            # "Expand to add\nmore events"
            n426 = Unbundle By Name(w1017) -> ("Self"=w1014:refnum<class "Setting Database.lvclass">)
            n427 = call <vilib>:"GetProtectedEvents.vi"("SMO"=w1014) -> ("error out"=w1021:errorcluster, "SMO Protected Events"=w1015:T19)  [unwired: 8 in, 1 out]
            n428 = call "Setting Database.GetPrivateEvents.vi"("Setting Database"=w1014) -> ("error out"=w1020:errorcluster, "Private Events"=w1013:T20)  [unwired: 8 in, 1 out]
            n429 = register-events(w1015, w1013) -> (reference out=w1016:refnum<event-registration>, error out=w1022:errorcluster)  [unwired: 2 in]
            n430 = Merge Errors(w1024, w1022, w1021, w1020) -> (w1023:errorcluster)
            n431 = call <vilib>:"Add State(s) to Queue__jki_lib_state_machine.vi"("State(s) in (\"\")"=w1019) -> ("States Out"=w1018:string)  [unwired: 14 in]
          }
          frame "Events: Unregister" {
            n432 = Unregister For Events(event registration refnum=w1025, error in=w1030) -> (error out=w1029:errorcluster)
            n433 = call <vilib>:"Clear Errors.vi"("error in (no error)"=w1029) -> ()  [unwired: 5 in, 2 out]
            n434 = call <vilib>:"Add State(s) to Queue__jki_lib_state_machine.vi"("State(s) in (\"\")"=w1028) -> ("States Out"=w1027:string)  [unwired: 14 in]
          }
          frame "---------- Publish ----------" {
            n435 = Unbundle By Name(w1032) -> ("Self"=w1031:refnum<class "Setting Database.lvclass">)
            n436 = Bundle By Name(cluster=w1032, "Self"=w1031) -> (w1033:T6)
            n437 = call <vilib>:"Add State(s) to Queue__jki_lib_state_machine.vi"("State(s) in (\"\")"=w1036) -> ("States Out"=w1035:string)  [unwired: 14 in]
          }
          frame "Publish: Active Funnel" {
            n438 = Unbundle By Name(w1045) -> ("Self"=w1044:refnum<class "Setting Database.lvclass">)
            n439 = call "Read Active Funnel.vi"("error in (no error)"=w1038, "Setting Database in"=w1044) -> ("error out"=w1040:errorcluster, "Active Funnel"=w1041:refnum<class "Funnel Settings.lvclass">, "Setting Database out"=w1043:refnum<class "Setting Database.lvclass">)  [unwired: 7 in]
            n440 = call "Setting Database.NewActiveFunnel.vi"("error in (no error)"=w1040, "NewActiveFunnel"=w1041, "Setting Database"=w1043) -> ("error out"=w1039:errorcluster, "Setting Database"=w1042:refnum<class "Setting Database.lvclass">)  [unwired: 7 in]
            n441 = Bundle By Name(cluster=w1045, "Self"=w1042) -> (w1046:T6)
            n442 = call <vilib>:"Add State(s) to Queue__jki_lib_state_machine.vi"("State(s) in (\"\")"=w1049) -> ("States Out"=w1048:string)  [unwired: 14 in]
          }
          frame "Publish: Funnels" {
            n443 = Unbundle By Name(w1057) -> ("Self"=w1056:refnum<class "Setting Database.lvclass">)
            n444 = call "Read Funnels.vi"("error in (no error)"=w1050, "Setting Database in"=w1056) -> ("error out"=w1052:errorcluster, "Funnels"=w1053:refnum<class "Funnel Settings.lvclass">[], "Setting Database out"=w1055:refnum<class "Setting Database.lvclass">)  [unwired: 7 in]
            n445 = call "Setting Database.FunnelsUpdated.vi"("error in (no error)"=w1052, "FunnelsUpdated"=w1053, "Setting Database"=w1055) -> ("error out"=w1051:errorcluster, "Setting Database out"=w1054:refnum<class "Setting Database.lvclass">)  [unwired: 7 in]
            n446 = Bundle By Name(cluster=w1057, "Self"=w1054) -> (w1058:T6)
            n447 = call <vilib>:"Add State(s) to Queue__jki_lib_state_machine.vi"("State(s) in (\"\")"=w1061) -> ("States Out"=w1060:string)  [unwired: 14 in]
          }
          frame "Publish: Active Dot" {
            n448 = Unbundle By Name(w1069) -> ("Self"=w1068:refnum<class "Setting Database.lvclass">)
            n449 = call "Read Active Dot.vi"("error in (no error)"=w1067, "Setting Database in"=w1068) -> ("error out"=w1064:errorcluster, "Active Dot"=w1062:refnum<class "Dot Settings.lvclass">, "Setting Database out"=w1066:refnum<class "Setting Database.lvclass">)  [unwired: 7 in]
            n450 = call "Setting Database.NewActiveDot.vi"("error in (no error)"=w1064, "NewActiveDot"=w1062, "Setting Database"=w1066) -> ("error out"=w1063:errorcluster, "Setting Database"=w1065:refnum<class "Setting Database.lvclass">)  [unwired: 7 in]
            n451 = Bundle By Name(cluster=w1069, "Self"=w1065) -> (w1070:T6)
            n452 = call <vilib>:"Add State(s) to Queue__jki_lib_state_machine.vi"("State(s) in (\"\")"=w1073) -> ("States Out"=w1072:string)  [unwired: 14 in]
          }
          frame "Publish: Dots" {
            n453 = Unbundle By Name(w1081) -> ("Self"=w1079:refnum<class "Setting Database.lvclass">)
            n454 = call "Read Dots.vi"("error in (no error)"=w1080, "Setting Database in"=w1079) -> ("error out"=w1075:errorcluster, "Dots"=w1074:refnum<class "Dot Settings.lvclass">[], "Setting Database out"=w1078:refnum<class "Setting Database.lvclass">)  [unwired: 7 in]
            n455 = call "Setting Database.DotsUpdated.vi"("error in (no error)"=w1075, "DotsUpdated"=w1074, "Setting Database"=w1078) -> ("error out"=w1076:errorcluster, "Setting Database out"=w1077:refnum<class "Setting Database.lvclass">)  [unwired: 7 in]
            n456 = Bundle By Name(cluster=w1081, "Self"=w1077) -> (w1082:T6)
            n457 = call <vilib>:"Add State(s) to Queue__jki_lib_state_machine.vi"("State(s) in (\"\")"=w1085) -> ("States Out"=w1084:string)  [unwired: 14 in]
          }
          frame "Publish: Active Rectangle" {
            n458 = Unbundle By Name(w1093) -> ("Self"=w1089:refnum<class "Setting Database.lvclass">)
            n459 = call "Read Active Rectangle.vi"("error in (no error)"=w1086, "Setting Database in"=w1089) -> ("error out"=w1090:errorcluster, "Active Rectangle"=w1091:refnum<class "Rectangle Settings.lvclass">, "Setting Database out"=w1092:refnum<class "Setting Database.lvclass">)  [unwired: 7 in]
            n460 = call "Setting Database.NewActiveRectangle.vi"("error in (no error)"=w1090, "NewActiveRectangle"=w1091, "Setting Database"=w1092) -> ("error out"=w1087:errorcluster, "Setting Database"=w1088:refnum<class "Setting Database.lvclass">)  [unwired: 7 in]
            n461 = Bundle By Name(cluster=w1093, "Self"=w1088) -> (w1094:T6)
            n462 = call <vilib>:"Add State(s) to Queue__jki_lib_state_machine.vi"("State(s) in (\"\")"=w1097) -> ("States Out"=w1096:string)  [unwired: 14 in]
          }
          frame "Publish: Rectangles" {
            n463 = Unbundle By Name(w1105) -> ("Self"=w1103:refnum<class "Setting Database.lvclass">)
            n464 = call "Read Rectangles.vi"("error in (no error)"=w1098, "Setting Database in"=w1103) -> ("error out"=w1101:errorcluster, "Rectangles"=w1100:refnum<class "Rectangle Settings.lvclass">[], "Setting Database out"=w1102:refnum<class "Setting Database.lvclass">)  [unwired: 7 in]
            n465 = call "Setting Database.RectanglesUpdated.vi"("error in (no error)"=w1101, "RectanglesUpdated"=w1100, "Setting Database"=w1102) -> ("error out"=w1099:errorcluster, "Setting Database out"=w1104:refnum<class "Setting Database.lvclass">)  [unwired: 7 in]
            n466 = Bundle By Name(cluster=w1105, "Self"=w1104) -> (w1106:T6)
            n467 = call <vilib>:"Add State(s) to Queue__jki_lib_state_machine.vi"("State(s) in (\"\")"=w1109) -> ("States Out"=w1108:string)  [unwired: 14 in]
          }
          frame "Publish: Active Path" {
            n468 = Unbundle By Name(w1111) -> ("Self"=w1115:refnum<class "Setting Database.lvclass">)
            n469 = call "Read Active Path.vi"("error in (no error)"=w1119, "Setting Database in"=w1115) -> ("error out"=w1121:errorcluster, "Path Settings.lvclass"=w1113:refnum<class "Path Settings.lvclass">, "Setting Database out"=w1114:refnum<class "Setting Database.lvclass">)  [unwired: 7 in]
            n470 = call "Setting Database.NewActivePath.vi"("error in (no error)"=w1121, "NewCurrentPath"=w1113, "Setting Database"=w1114) -> ("error out"=w1120:errorcluster, "Setting Database"=w1110:refnum<class "Setting Database.lvclass">)  [unwired: 7 in]
            n471 = Bundle By Name(cluster=w1111, "Self"=w1110) -> (w1112:T6)
            n472 = call <vilib>:"Add State(s) to Queue__jki_lib_state_machine.vi"("State(s) in (\"\")"=w1118) -> ("States Out"=w1117:string)  [unwired: 14 in]
          }
          frame "Publish: Paths" {
            n473 = Unbundle By Name(w1127) -> ("Self"=w1124:refnum<class "Setting Database.lvclass">)
            n474 = call "Read Paths.vi"("error in (no error)"=w1131, "Setting Database in"=w1124) -> ("error out"=w1133:errorcluster, "Paths"=w1122:refnum<class "Path Settings.lvclass">[], "Setting Database out"=w1123:refnum<class "Setting Database.lvclass">)  [unwired: 7 in]
            n475 = call "Setting Database.PathsUpdated.vi"("error in (no error)"=w1133, "PathsUpdated"=w1122, "Setting Database"=w1123) -> ("error out"=w1132:errorcluster, "Setting Database out"=w1125:refnum<class "Setting Database.lvclass">)  [unwired: 7 in]
            n476 = Bundle By Name(cluster=w1127, "Self"=w1125) -> (w1126:T6)
            n477 = call <vilib>:"Add State(s) to Queue__jki_lib_state_machine.vi"("State(s) in (\"\")"=w1130) -> ("States Out"=w1129:string)  [unwired: 14 in]
          }
        }
      }
    }
    frame Error {
    }
  }
  n478 = call-parent "Process.vi"("error in"=w8, "SMO"=w4) -> ("error out"=w7:errorcluster, "SMO out"=→"Setting Database out":refnum<class "Setting Database.lvclass">)  [unwired: 8 in]
  n479 = Merge Errors(w7, w6) -> (→"error out":errorcluster)
